vi "Traffic Monitoring Hub.vi"() -> ()   [LabVIEW 2018]
uses:
  TrafficMap/TrafficMap.lvclass
  <vilib>/LabVIEW Open Source Project/MQTT Broker/Client/Client.lvclass
  C:/Program Files (x86)/National Instruments/LabVIEW 2018/vi.lib/LabVIEW Open Source Project/MQTT Broker/MQTT_Base/MQTT_Base.lvclass
  <vilib>/LabVIEW Open Source Project/MQTT Broker/Control Packets/PUBLISH/PUBLISH.lvclass
  C:/Program Files (x86)/National Instruments/LabVIEW 2018/vi.lib/LabVIEW Open Source Project/MQTT Broker/Control Packets/ControlPacket/ControlPacket.lvclass
  typedefs/Node Type -- enum.ctl
  CarPool/CarPool.lvclass
  Zone/Zone.lvclass/Zone.ctl
  typedefs/RequestPayload -- cluster.ctl
  <vilib>/LabVIEW Open Source Project/MQTT Broker/Control Packets/ControlPacket/ControlPacket.lvclass/ControlPacket.ctl
  typedefs/ResponsePayload -- cluster.ctl
  TrafficMap/TrafficMap.lvclass/TrafficMap.ctl
  Car/Car State -- enum.ctl
  Car/Car.lvclass/Car.ctl
  Serializer.JKI-JSON/Serializer.JKI-JSON.lvclass
  C:/Program Files (x86)/National Instruments/LabVIEW 2018/vi.lib/LabVIEW Open Source Project/Serializer/Serializer/Serializer.lvclass
  <vilib>/LabVIEW Open Source Project/MQTT Broker/MQTT_Base/MQTT_Base.lvclass/MQTT_Base.ctl
  <vilib>/LabVIEW Open Source Project/MQTT Broker/Client/Client.lvclass/Client.ctl
  <vilib>/LabVIEW Open Source Project/MQTT Broker/Control Packets/CONNECT/ConnectFlags -- cluster.ctl
  typedefs/DisconnectPayload-- cluster.ctl
  typedefs/WillPayload -- cluster.ctl
  typedefs/ConnectPayload-- cluster.ctl
  82f4286b-0a94-4b9a-b9d4-821bcdb1e953.vi
  0d705227-134d-4031-8d1e-e35da49b8ba8.vi
  3d3687d4-2784-4a3f-94ff-e25152285f29.vi
  38838a55-6234-4be0-b764-729cd2a94195.vi
  e5968ec8-ddc8-4f80-9081-17407ede201a.vi
  bcdb7536-3eda-440d-b728-4c0836012992.vi
  bdf30a18-8ec8-4ac2-babb-b5048eb54a3e.vi
  3e129768-4a02-4394-80d2-37f91f557ee1.vi
  91350af8-47c3-4bac-a32d-49938f55f876.vi
  <vilib>/LabVIEW Open Source Project/Serializer/Serializer.FlattenedString/Serializer.FlattenedString.lvclass
  <vilib>/LabVIEW Open Source Project/MQTT Broker/MQTT_Base/Decode Publish Package.vi
  <vilib>/LabVIEW Open Source Project/Serializer/Serializer/Serializer.lvclass
  <vilib>/LabVIEW Open Source Project/MQTT Broker/MQTT_Base/MQTT_Base.lvclass
  <vilib>/LabVIEW Open Source Project/MQTT Broker/Control Packets/ControlPacket/ControlPacket.lvclass
  <vilib>/LabVIEW Open Source Project/MQTT Broker/Control Packets/CONNECT/CONNECT.lvclass
  <vilib>/addons/_JKI.lib/Serialization/JSON/JKI JSON Serialization.lvlib
  Car/Car.lvclass
  Zone/Zone.lvclass
  <vilib>/ptbypt/NI_PtbyPt.lvlib
panel:
  out "Zones":u32[](array[slide]) scale=0.0..11.4
  in  "# Cars":i32=1 min=1 max=20
  out "Message Frequency (Hz)":dbl
  out "error out":errorcluster
  out "Messages Processed":u32
  in  "Destroy Sim Cars":bool
  in  "Generate Sim Cars":bool
  out "Last Incoming Message":string
  out "Hub status":string
  out "Connection Status":string="Disconnected"
  out "Map":u16[][](graph)
  out "Zones":string[](array[string])
  in  "List Zones":bool
  out "Raw Packet String":string
  out "Payload":variant
  out "Topic":string
  # "Traffic Monitoring Hub"
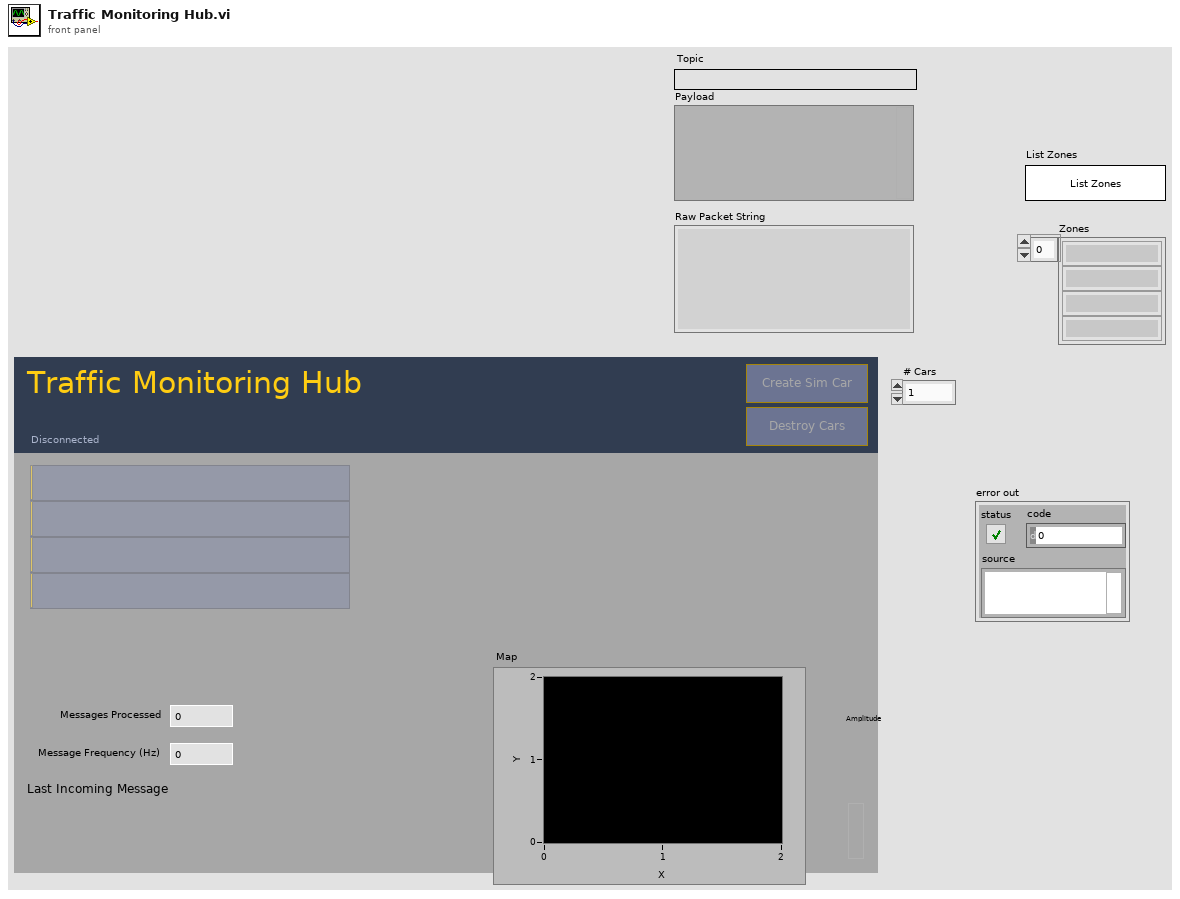
[diagram p1: front panel]
types:
  T1 = enum32{"Invalid", "Standard", "Closed", "Hidden", "Minimized", "Maximized"}
  T2 = enum32{"invalid app kind", "Development System", "Run Time System", "Student Edition", "Embedded LabVIEW", "Evaluation", "Custom"}
  T3 = typedef "RequestPayload -- cluster.ctl" = cluster{"request":string, "reply-to":string}
  T4 = typedef "ResponsePayload -- cluster.ctl" = cluster{"request":string, "reply":variant}
  T5 = typedef "Car.lvclass/Car State -- enum.ctl" = enum16{"parked", "driving"}
  T6 = typedef "CONNECT.lvclass/ConnectFlags -- cluster.ctl" = cluster{"Reserved":bool, "Clean Session":bool, "Will Flag":bool, "Will QoS 1":bool, "Will QoS 2":bool, "Will Retain":bool, "Password Flag":bool, "User Name Flag":bool}
  T7 = cluster{"Will Topic":string, "Will Message":string, "Username":string, "Password":string}
  T8 = typedef "DisconnectPayload-- cluster.ctl" = cluster{"timestamp":string}
  T9 = typedef "WillPayload -- cluster.ctl" = cluster{"message":string}
  T10 = typedef "ConnectPayload-- cluster.ctl" = cluster{"Node type":string}
  T11 = typedef "Node Type -- enum.ctl" = enum16{"Car", "Hub", "Sensor", "Relay"}
  T12 = cluster{"Core":cluster{"Current VI Reference":refnum<vi>, "Close Panel on Exit?":bool}, "server address":string, "project namespace":string, "Client Name":string, "Node type":T11, "Client":refnum<class "Client.lvclass">, "Close on MQTT Disconnection?":bool, "Subscription":string, "AppMessage":refnum<class "PUBLISH.lvclass">, "stop signal":refnum<user-event>, "TrafficMap":refnum<class "TrafficMap.lvclass">, "CarPool":refnum<class "CarPool.lvclass">, "Clones":string[]}
  T13 = cluster{"Current VI Reference":refnum<vi>, "Close Panel on Exit?":bool}
  T14 = cluster{"Messages Processed":u32, "seconds since 1Jan1904":timestamp}
  T15 = cluster{"Messages Processed":u32, "seconds since 1Jan1904":dbl}
  T16 = typedef "MQTT Server.lvlib/Client.lvclass/Public Events -- cluster.ctl" = cluster{"Connection Status":refnum<user-event>, "Connected":refnum<user-event>, "Application Message":refnum<user-event>}
  T17 = typedef "ControlPacket.lvclass/QualityOfService -- enum.ctl" = enum16{"0 (At Most Once)", "1 (At Least Once)", "2 (Exactly Once)"}
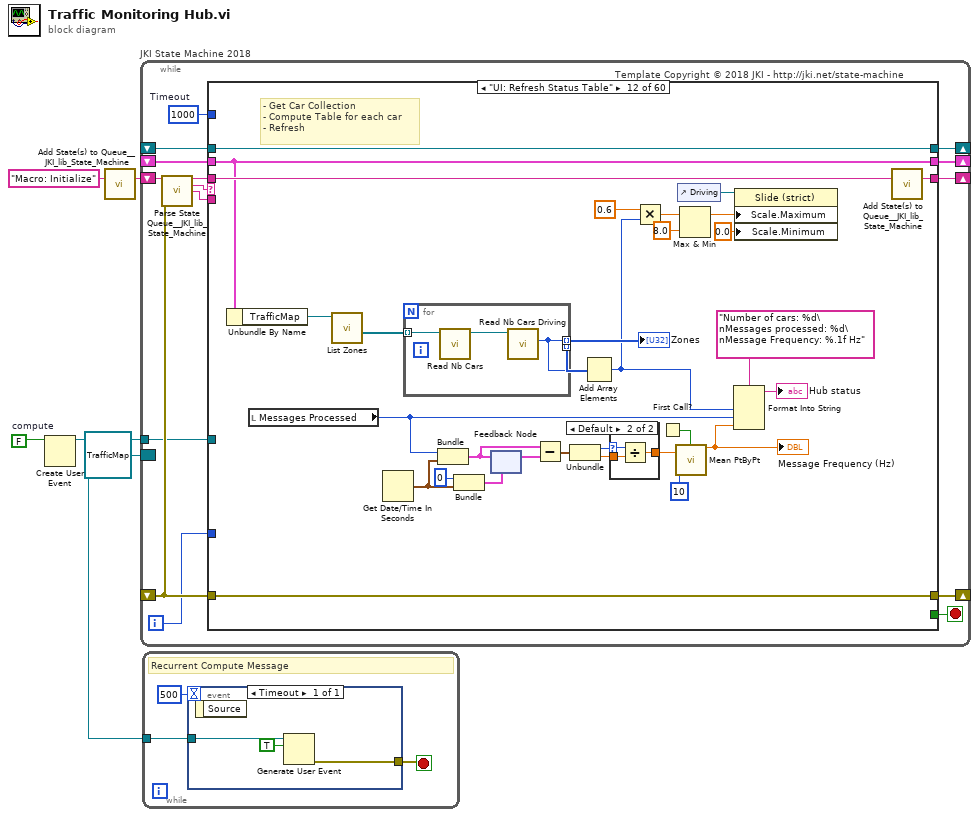
[diagram p0: block diagram]
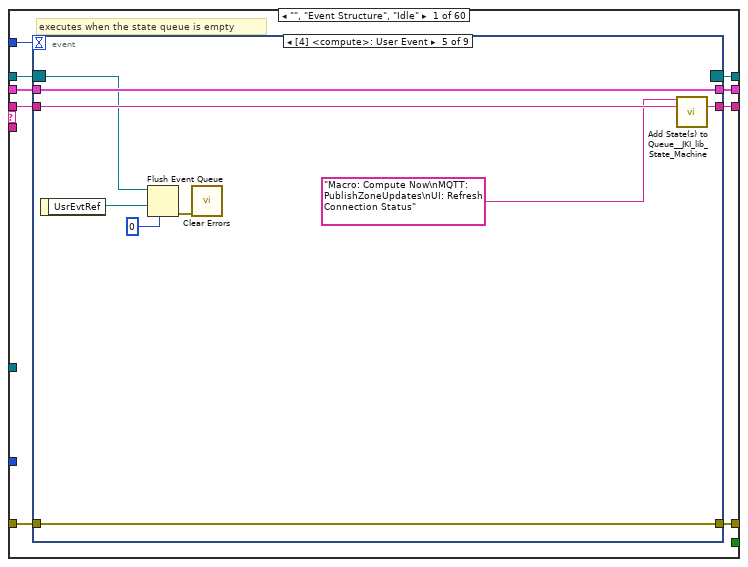
[diagram p2: hidden frame]
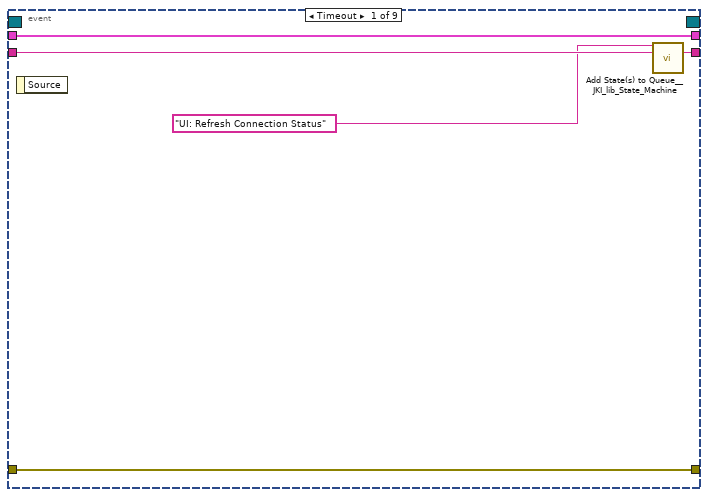
[diagram p3: hidden frame]
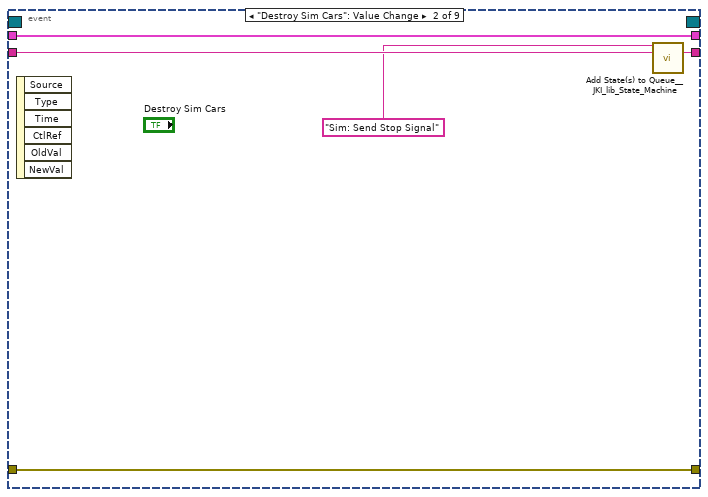
[diagram p4: hidden frame]
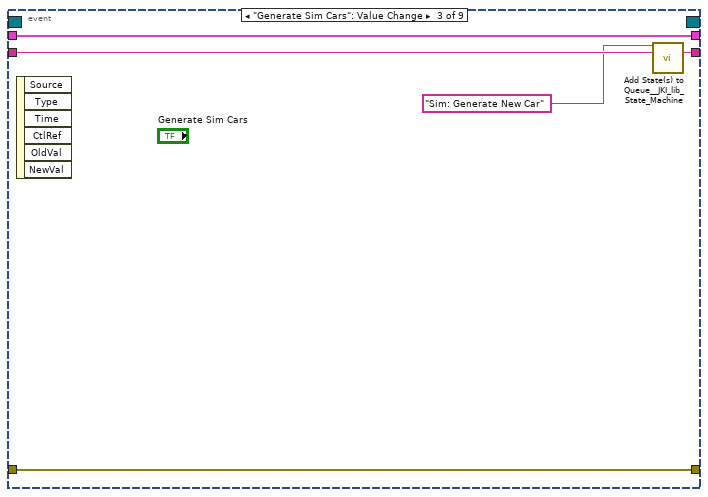
[diagram p5: hidden frame]
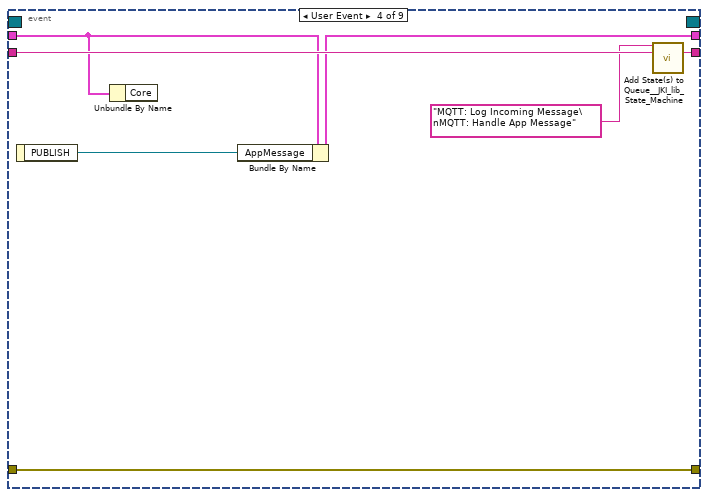
[diagram p6: hidden frame]
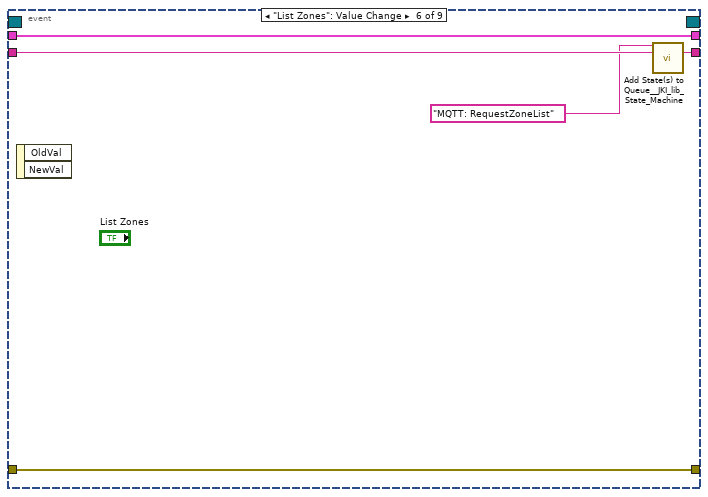
[diagram p7: hidden frame]
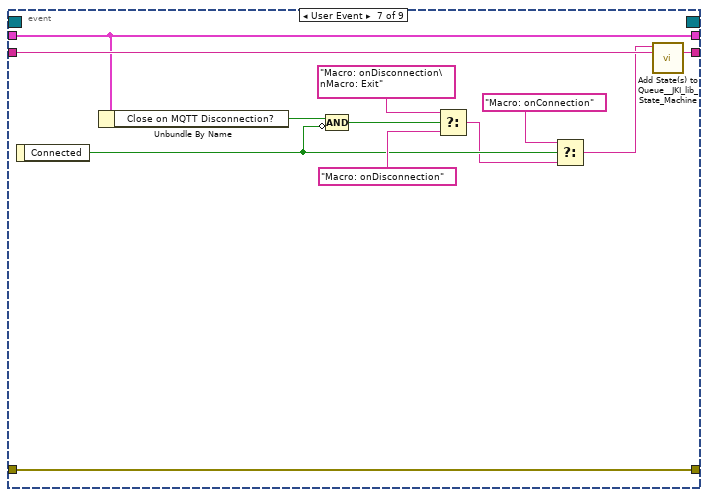
[diagram p8: hidden frame]
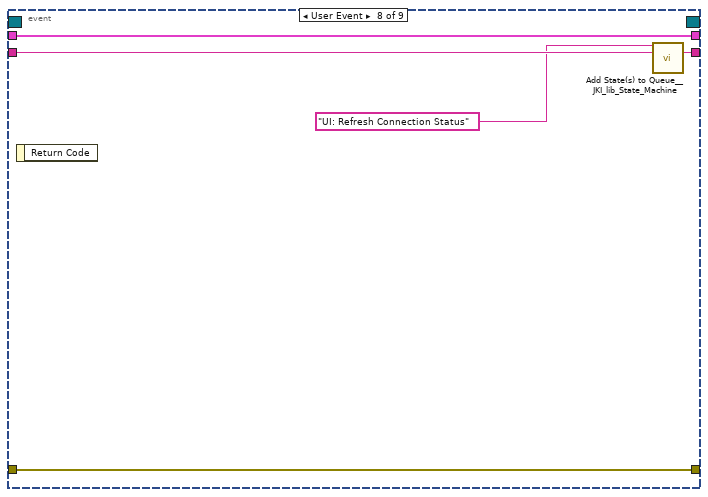
[diagram p9: hidden frame]
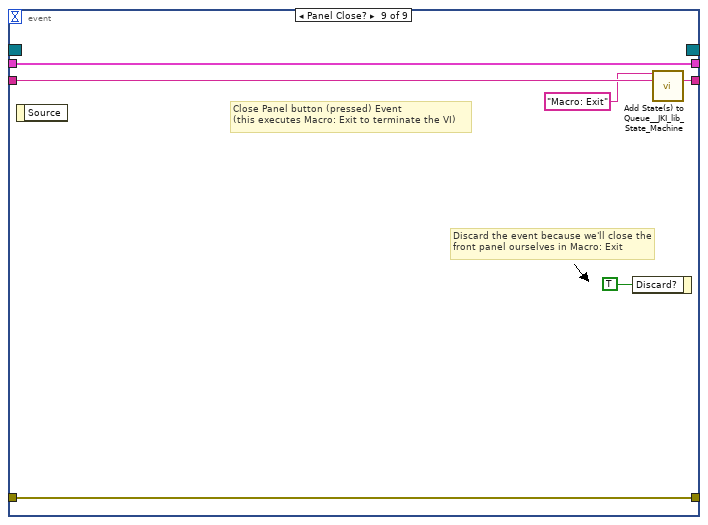
[diagram p10: hidden frame]
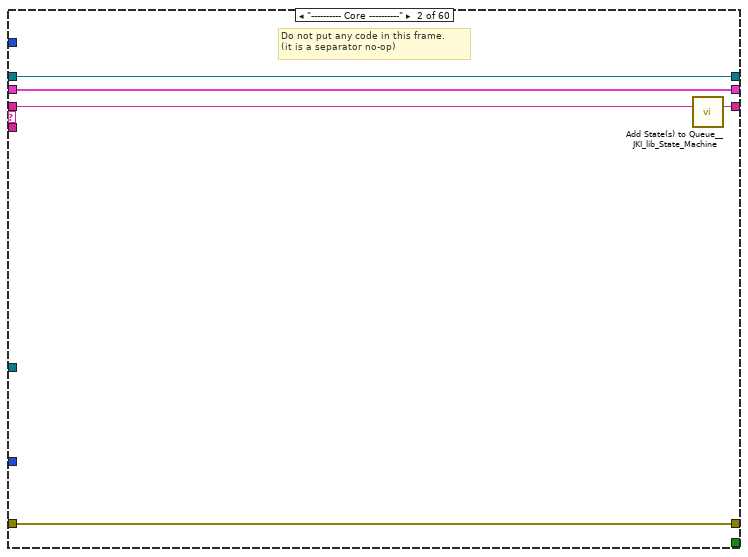
[diagram p11: hidden frame]
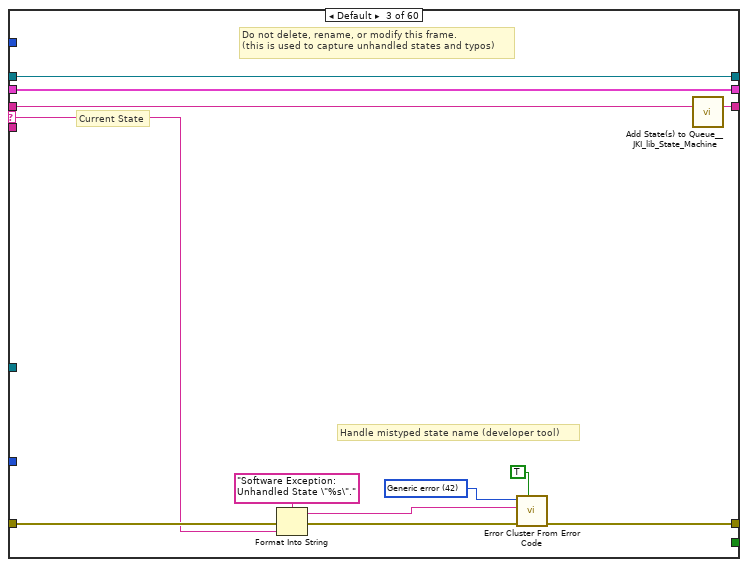
[diagram p12: hidden frame]
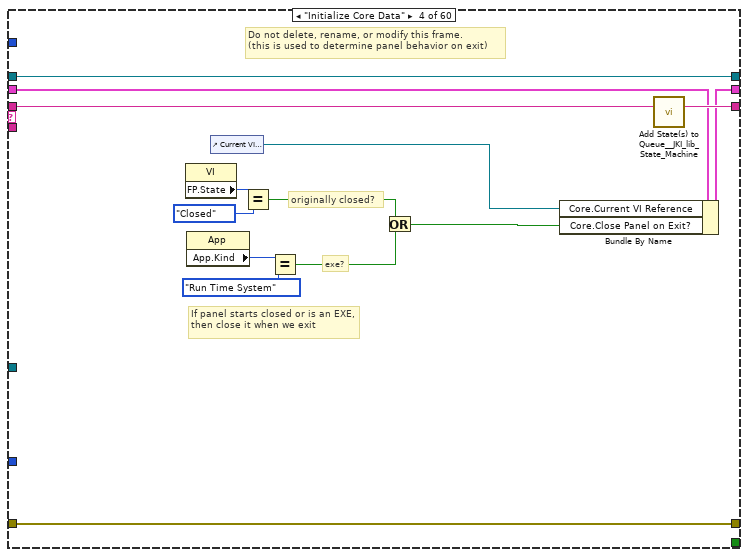
[diagram p13: hidden frame]
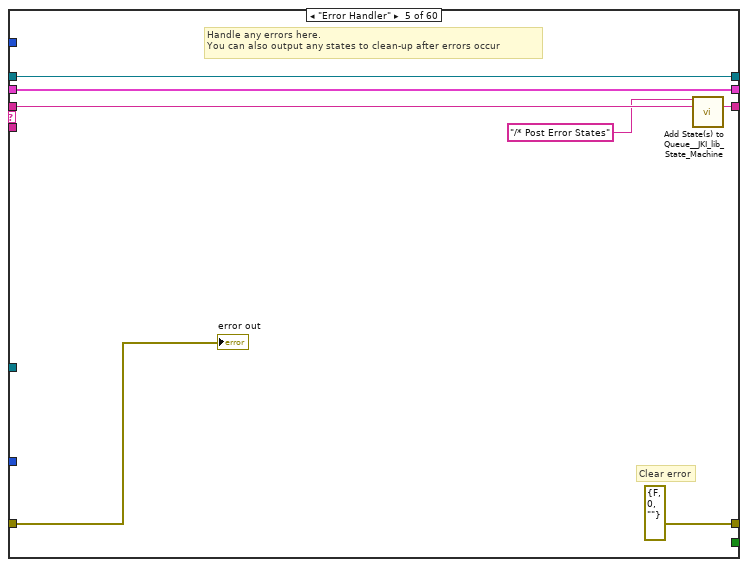
[diagram p14: hidden frame]
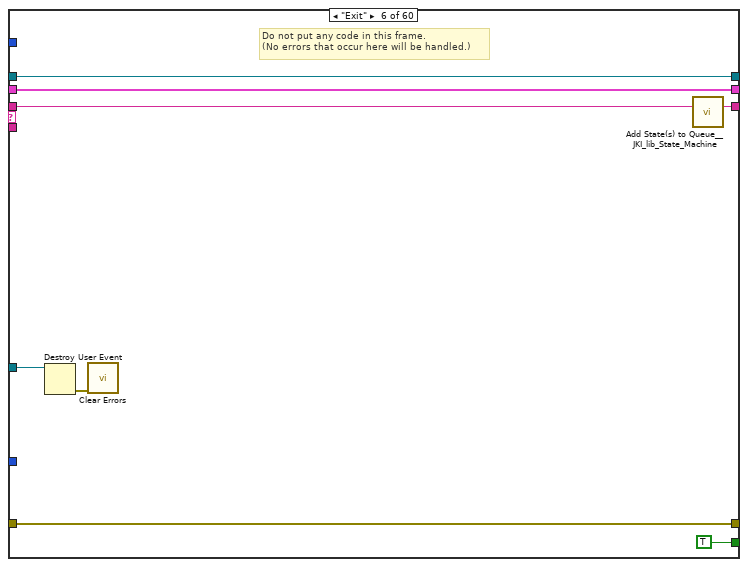
[diagram p15: hidden frame]
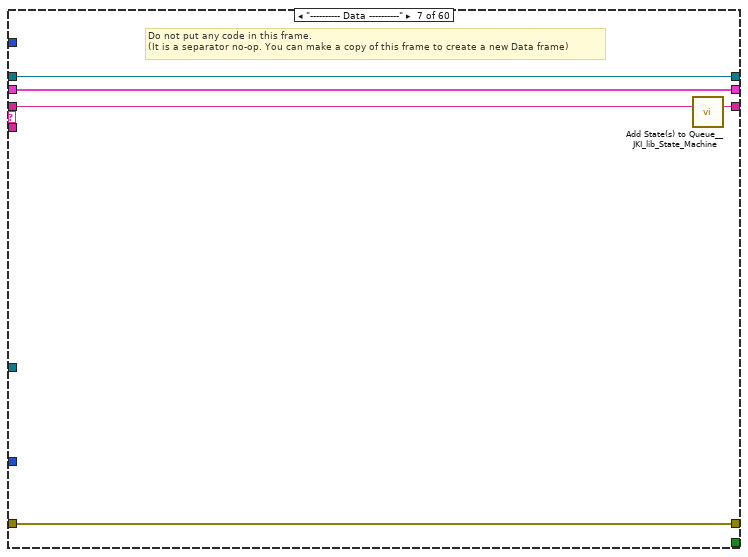
[diagram p16: hidden frame]
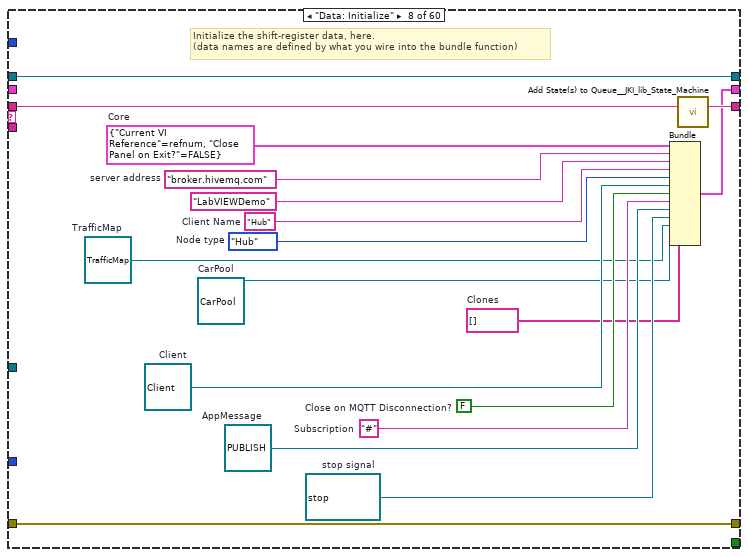
[diagram p17: hidden frame]
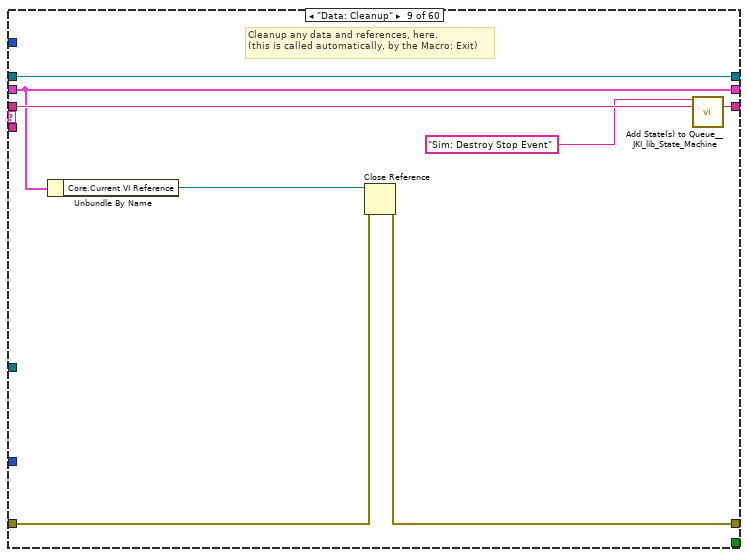
[diagram p18: hidden frame]
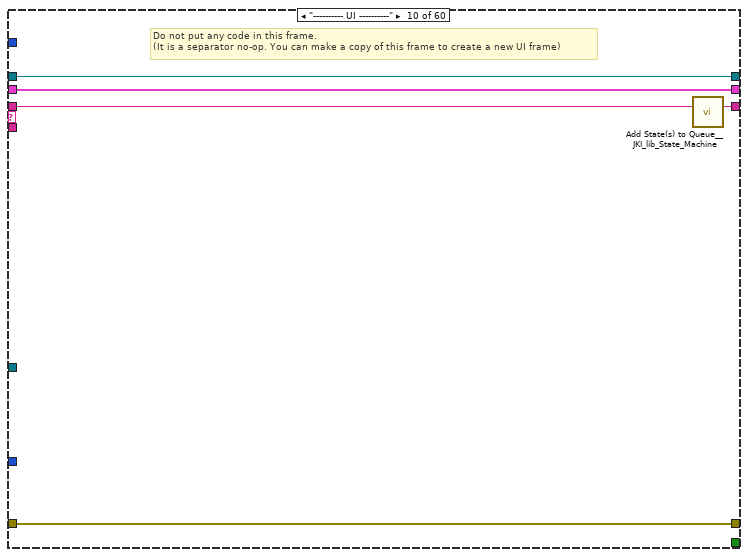
[diagram p19: hidden frame]
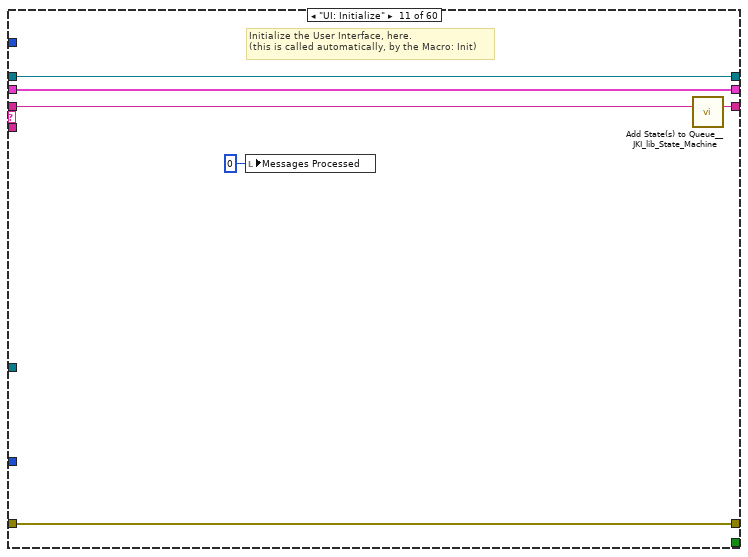
[diagram p20: hidden frame]
diagram:
  w3 = FALSE  # compute
  n1 = Create User Event(user event datatype=w3) -> (user event=w2:refnum<user-event>)  [unwired: 1 in, 1 out]
  n2 = call <vilib>:"Add State(s) to Queue__JKI_lib_State_Machine.vi"("State(s) in (\"\")"="Macro: Initialize") -> ("States Out"=w5:string)  [unwired: 14 in]
  n3 = while "JKI State Machine 2018" {
    shift-right: [w13] -> _
    shift-left: _ -> [w12]
    shift-right: [w16] -> _
    shift-left: _ -> [w10]
    shift-right: [w15] -> _
    shift-left: w5 -> [w17]
    shift-right: [w8] -> _
    shift-left: _ -> [w9]
    tunnel: w2 -> [w7]
    border: refnum<class "TrafficMap.lvclass"> refnum ("TrafficMap out") -> [_]
    i -> [w6]
    stop <- w14 stop-if-true
    w11 = 1000  # Timeout
    # "Template Copyright © 2018 JKI - http://jki.net/state-machine"
    n4 = call <vilib>:"Parse State Queue__JKI_lib_State_Machine.vi"("State Queue"=w17, "Error In (no error)"=w10) -> ("Remaining States"=w19:string, "Current State"=w20:string, "Arguments"=w18:string)  [unwired: 11 in]
    n5 = case shown="\"UI: Refresh Status Table\"" w20 {
      selector: w20 -> [_ _ w95 _ _ _ _ _ _ _ _ _ _ _ _ _ _ _ _ _ _ _ _ _ _ _ _ _ _ _ _ _ _ _ _ _ _ _ _ _ _ _ _ _ _ _ _ _ _ _ _ _ _ _ _ _ _ _ _ _]
      tunnel: w19 -> [w29 w93 w99 w119 w126 w134 w139 w157 w165 w170 w176 w207 w226 w233 w245 w315 w321 w327 w333 w339 w345 w351 w357 w363 w368 w374 w388 w393 w401 w407 w416 w431 w449 w466 w485 w493 w516 w540 w545 w557 w569 w593 w604 w617 w630 w644 w660 w724 w753 w779 w802 w817 w870 w884 w895 w926 w942 w953 w959 w966]
      tunnel: w18 -> [_ _ _ _ _ _ _ _ _ _ _ _ _ w228 w239 _ _ _ _ _ _ _ _ _ _ _ _ _ _ _ _ _ _ _ _ _ _ _ _ _ _ _ _ _ _ _ _ _ _ _ _ _ _ _ _ _ _ _ _ _]
      tunnel: w12 -> [w27 w90 w97 w112 w123 w132 w136 _ w160 w167 w174 w203 w216 w231 w241 w312 w318 w324 w330 w336 w342 w348 w354 w360 w365 w371 w385 w390 w395 w403 w410 w421 w446 w451 w482 w487 w511 w536 w542 w555 w566 w590 w597 w614 w627 w641 w645 w721 w750 w776 w799 w807 w867 w881 w888 w923 w939 w950 w954 w964]
      tunnel: [w26 w91 w101 w116 errorcluster {"status"=FALSE, "code"=0, "source"=""} ("error out") w131 w137 w154 w161 w168 w173 w205 w224 w229 w242 w313 w319 w325 w331 w337 w343 w349 w355 w361 w366 w372 w386 w391 w399 w405 w414 w429 w447 w460 w483 w491 w514 w538 w543 w547 w559 w584 w594 w606 w622 w632 w657 w719 w748 w774 w797 w814 w860 w874 w885 w914 w930 w945 w955 w961] -> w16
      tunnel: w10 -> [w25 w91 w100 w116 w120 w131 w137 w154 w162 w168 w173 w205 w224 w230 w243 w313 w319 w325 w331 w337 w343 w349 w355 w361 w366 w372 w386 w391 w399 w405 w414 w429 w447 w461 w483 w491 w514 w538 w543 w553 w562 w585 w595 w607 w623 w633 w657 w719 w748 w774 w797 w814 w861 w875 w886 w915 w931 w943 w956 w962]
      tunnel: [w28 w92 w98 w118 w125 w133 w138 w156 w164 w169 w175 w206 w225 w232 w244 w314 w320 w326 w332 w338 w344 w350 w356 w362 w367 w373 w387 w392 w400 w406 w415 w430 w448 w465 w484 w492 w515 w539 w544 w556 w568 w592 w603 w616 w629 w643 w659 w723 w752 w778 w801 w816 w869 w883 w894 w925 w941 w952 w958 w965] -> w15
      tunnel: [_ _ _ _ _ TRUE _ _ _ _ _ _ _ _ _ _ _ _ _ _ _ _ _ _ _ _ _ _ _ _ _ _ _ _ _ _ _ _ _ _ _ _ _ _ _ _ _ _ _ _ _ _ _ _ _ _ _ _ _ _] -> w14
      tunnel: [w24 w90 w97 w117 w123 w132 w136 w155 w160 w167 w174 w203 w216 w231 w241 w312 w318 w324 w330 w336 w342 w348 w354 w360 w365 w371 w385 w390 w394 w403 w409 w420 w446 w464 w482 w486 w510 w536 w542 w554 w567 w591 w597 w615 w628 w642 w645 w722 w751 w777 w800 w807 w868 w882 w888 w924 w940 w951 w954 w964] -> w13
      tunnel: w11 -> [w23 _ _ _ _ _ _ _ _ _ _ _ _ _ _ _ _ _ _ _ _ _ _ _ _ _ _ _ _ _ _ _ _ _ _ _ _ _ _ _ _ _ _ _ _ _ _ _ _ _ _ _ _ _ _ _ _ _ _ _]
      tunnel: w9 -> [w22 w89 w94 w106 w121 w129 w135 w148 w159 w166 w172 w204 w223 w227 w238 w311 w316 w322 w328 w334 w340 w346 w352 w358 w364 w369 w377 w389 w398 w404 w413 w428 w445 w463 w481 w490 w513 w537 w541 w552 _ w589 w602 w613 w626 w640 w658 w720 w749 w775 w798 w815 w866 w880 w893 w922 w938 w949 w957 w960]
      tunnel: [w21 w89 w94 w106 w121 w129 w135 w148 w159 w166 w172 w204 w223 w227 w238 w311 w316 w322 w328 w334 w340 w346 w352 w358 w364 w369 w377 w389 w398 w404 w413 w428 w445 w463 w481 w490 w513 w537 w541 w552 w561 w589 w602 w613 w626 w640 w658 w720 w749 w775 w798 w815 w866 w880 w893 w922 w938 w949 w957 w960] -> w8
      tunnel: w7 -> [_ _ _ _ _ w128 _ _ _ _ _ _ _ _ _ _ _ _ _ _ _ _ _ _ _ _ w375 _ _ _ _ _ _ _ _ _ _ _ _ _ w558 _ _ _ _ _ _ _ _ _ _ _ _ _ _ _ _ _ _ _]
      tunnel: w6 -> [_ _ _ _ _ _ _ _ _ _ _ _ _ _ _ _ _ _ _ _ _ _ _ _ _ _ _ _ _ _ _ _ _ _ _ _ w500 _ _ _ _ _ _ _ _ _ _ _ _ _ _ _ _ _ _ _ _ _ _ _]
      frame "", "Event Structure", "Idle" {
        # "executes when the state queue is empty"
        n6 = event shown="[4] <compute>: User Event" {
          selector: w22 -> [_ _ _ _ w55 _ _ _ _]
          dyn-events: [_ _ _ _ _ _ _ _ _] -> w21
          timeout: w23 -> [_ _ _ _ _ _ _ _ _]
          tunnel: w29 -> [w34 w39 w44 w51 w60 w65 w77 w82 w88]
          tunnel: [w33 w38 w43 w50 w59 w64 w76 w81 w87] -> w28
          tunnel: w27 -> [w32 w36 w41 w47 w56 w61 w74 w79 w85]
          tunnel: [w31 w37 w42 w49 w58 w63 w75 w80 w86] -> w26
          tunnel: w25 -> [w31 w37 w42 w49 w58 w63 w75 w80 w86]
          tunnel: [w32 w36 w41 w46 w56 w61 w74 w79 w85] -> w24
          event Timeout {
            n7 = event-data() -> ()  [unwired: 1 in, 1 out]
            n8 = call <vilib>:"Add State(s) to Queue__JKI_lib_State_Machine.vi"("State(s) in Front (\"\")"="UI: Refresh Connection Status", "State(s) in (\"\")"=w34) -> ("States Out"=w33:string)  [unwired: 13 in]
          }
          event "Destroy Sim Cars": Value Change {
            n9 = event-data() -> ()  [unwired: 1 in, 6 out]
            n10 = call <vilib>:"Add State(s) to Queue__JKI_lib_State_Machine.vi"("State(s) in Front (\"\")"="Sim: Send Stop Signal", "State(s) in (\"\")"=w39) -> ("States Out"=w38:string)  [unwired: 13 in]
          }
          event "Generate Sim Cars": Value Change {
            n11 = event-data() -> ()  [unwired: 1 in, 6 out]
            n12 = call <vilib>:"Add State(s) to Queue__JKI_lib_State_Machine.vi"("State(s) in Front (\"\")"="Sim: Generate New Car", "State(s) in (\"\")"=w44) -> ("States Out"=w43:string)  [unwired: 13 in]
          }
          event User Event {
            n13 = event-data() -> ("PUBLISH"=w48:refnum<class "PUBLISH.lvclass">)  [unwired: 1 in]
            n14 = Unbundle By Name(w47) -> ()  [unwired: 1 out]
            n15 = Bundle By Name(cluster=w47, "AppMessage"=w48) -> (w46:T12)
            n16 = call <vilib>:"Add State(s) to Queue__JKI_lib_State_Machine.vi"("State(s) in Front (\"\")"="MQTT: Log Incoming Message\nMQTT: Handle App Message", "State(s) in (\"\")"=w51) -> ("States Out"=w50:string)  [unwired: 13 in]
          }
          event User Event {
            n17 = event-data() -> ("UsrEvtRef"=w54:refnum<user-event>)  [unwired: 1 in]
            n18 = Flush Event Queue(0:w55, 2:w54, 5:0 ("keep most recent")) -> (11:w52:errorcluster)  [unwired: 3 in, 2 out]
            n19 = call <vilib>:"Clear Errors.vi"("error in (no error)"=w52) -> ()  [unwired: 5 in, 2 out]
            n20 = call <vilib>:"Add State(s) to Queue__JKI_lib_State_Machine.vi"("State(s) in Front (\"\")"="Macro: Compute Now\nMQTT: PublishZoneUpdates\nUI: Refresh Connection Status", "State(s) in (\"\")"=w60) -> ("States Out"=w59:string)  [unwired: 13 in]
          }
          event "List Zones": Value Change {
            n21 = event-data() -> ()  [unwired: 1 in, 2 out]
            n22 = call <vilib>:"Add State(s) to Queue__JKI_lib_State_Machine.vi"("State(s) in Front (\"\")"="MQTT: RequestZoneList", "State(s) in (\"\")"=w65) -> ("States Out"=w64:string)  [unwired: 13 in]
          }
          event User Event {
            n23 = event-data() -> ("Connected"=w69:bool)  [unwired: 1 in]
            n24 = Unbundle By Name(w74) -> ("Close on MQTT Disconnection?"=w73:bool)
            n25 = Compound Arithmetic op=AND(w73, invert w69) -> (w72:bool)
            n26 = Select(t="Macro: onDisconnection\nMacro: Exit", s=w72, f="Macro: onDisconnection" ("t")) -> (s? t:f=w67:string)
            n27 = Select(t="Macro: onConnection", s=w69, f=w67) -> (s? t:f=w66:string)
            n28 = call <vilib>:"Add State(s) to Queue__JKI_lib_State_Machine.vi"("State(s) in Front (\"\")"=w66, "State(s) in (\"\")"=w77) -> ("States Out"=w76:string)  [unwired: 13 in]
          }
          event User Event {
            n29 = event-data() -> ()  [unwired: 1 in, 1 out]
            n30 = call <vilib>:"Add State(s) to Queue__JKI_lib_State_Machine.vi"("State(s) in Front (\"\")"="UI: Refresh Connection Status", "State(s) in (\"\")"=w82) -> ("States Out"=w81:string)  [unwired: 13 in]
          }
          event Panel Close? {
            # "Discard the event because we'll close the front panel ourselves in Macro: Exit"
            # "Close Panel button (pressed) Event\n(this executes Macro: Exit to terminate the VI)"
            n31 = event-data() -> ()  [unwired: 1 in, 1 out]
            n32 = event-data("Discard?"=TRUE) -> ()  [unwired: 1 in, 1 out]
            n33 = call <vilib>:"Add State(s) to Queue__JKI_lib_State_Machine.vi"("State(s) in Front (\"\")"="Macro: Exit", "State(s) in (\"\")"=w88) -> ("States Out"=w87:string)  [unwired: 13 in]
          }
        }
      }
      frame "---------- Core ----------" {
        # "Do not put any code in this frame.\n(it is a separator no-op)"
        n34 = call <vilib>:"Add State(s) to Queue__JKI_lib_State_Machine.vi"("State(s) in (\"\")"=w93) -> ("States Out"=w92:string)  [unwired: 14 in]
      }
      frame Default {
        w104 = 42 items=["No error", "Argument error", "Memory is full", "Out of zone", "End of file", "File already open", "Generic file I/O error", "File not found", "File permission error", "Disk is full", "Duplicate path", "Too many files open", "System feature not enabled", "Resource file not found", "Cannot add resource", "Resource not found", "Image not found", "Image memory error", "Pen does not exist", "Config type invalid", "Config token not found", "Config parse error", "Config memory error", "Bad external code format", "Bad external code offset", "External code not present", "Null window", "Destroy window error", "Null menu", "Print aborted", "Bad print record", "Print driver error", "Windows error during printing", "Memory error during printing", "Print dialog error", "Generic print error", "Invalid device refnum", "Device not found", "Device parameter error", "Device unit error", "Cannot open device", "Device call aborted", "Generic error", "Cancelled by user", "Object ID too low", "Object ID too high", "Object not in heap", "Unknown heap", "Unknown object (invalid DefProc)", "Unknown object (DefProc not in table)", "Message out of range", "Invalid (null) method", "Unknown message", "Manager call not supported", "Bad address", "Network operation in progress", "Network operation timed out", "Connection is busy", "Network attribute not supported", "Network error", "Address in use", "System out of memory", "Connection aborted", "Connection refused", "Not connected", "Already connected", "Connection closed", "Initialization error (interapplication manager)", "Bad occurrence", "Wait on unbound occurrence handler", "Occurrence queue overflow", "Datalog type conflict", "Unused", "Unrecognized type (interapplication manager)", "Memory corrupt", "Failed to make temporary DLL", "Old CIN version", "Drag socket not found", "Failed to load drop-object", "Failed to register OLE object", "Failed to release OLE object", "Format specifier type mismatch", "Unknown format specifier", "Too few format specifiers", "Too many format specifiers", "Scan failed", "Newer CIN version", "Error converting to variant", "Runtime menu error", "Password tampered", "Variant attribute not found", "Incompatible variant data type", "Event data is not available", "Event Store is not present", "Occurrence is not found", "Event Queue is not created", "Event info is not available", "Refnum passed is NULL", "Error retrieving Class GUID", "Error retrieving CoClass GUID", "Error retrieving TypeLib GUID.", "Bad built application magic bytes.", "Specific driver is different from the specific driver associated with the Logical Name.", "There is no session opened to the class driver.", "Max Error", "MAX - Error with config objects", "MAX - Error loading configuration", "MAX - Group not supported"]
        # "Current State"
        # "Do not delete, rename, or modify this frame.\n(this is used to capture unhandled states and typos)"
        # "Handle mistyped state name (developer tool)"
        n35 = Format Into String(format string="Software Exception: Unhandled State \"%s\"." ("message"), error in=w100, w95) -> (resulting string=w103:string, error out=w102:errorcluster)  [unwired: 1 in]
        n36 = call <vilib>:"Error Cluster From Error Code.vi"("show call chain? (False)"=TRUE, "error in (no error)"=w102, "error message (\"\")"=w103, "error code (0)"=w104) -> ("error out"=w101:errorcluster)  [unwired: 5 in]
        n37 = call <vilib>:"Add State(s) to Queue__JKI_lib_State_Machine.vi"("State(s) in (\"\")"=w99) -> ("States Out"=w98:string)  [unwired: 14 in]
      }
      frame "Initialize Core Data" {
        # "Do not delete, rename, or modify this frame.\n(this is used to determine panel behavior on exit)"
        # "originally closed?"
        # "exe?"
        # "If panel starts closed or is an EXE, then close it when we exit"
        n38 = property class="VI"() -> ("FP.State"=w109:T1)  [unwired: 2 in, 2 out]
        n39 = property class="App"() -> ("App.Kind"=w115:T2)  [unwired: 2 in, 2 out]
        n40 = control-ref of="Current VI Reference"() -> (w110:refnum<vi>)
        n41 = Equal?(x=w109, y=T1."Closed" ("Front Panel Window:State")) -> (x = y?=w107:bool)
        n42 = Equal?(x=w115, y=T2."Run Time System" ("Application:Kind")) -> (x = y?=w113:bool)
        n43 = Or(x=w107, y=w113) -> (x .or. y?=w111:bool)
        n44 = Bundle By Name(cluster=w112, "Core.Current VI Reference"=w110, "Core.Close Panel on Exit?"=w111) -> (w117:T12)
        n45 = call <vilib>:"Add State(s) to Queue__JKI_lib_State_Machine.vi"("State(s) in (\"\")"=w119) -> ("States Out"=w118:string)  [unwired: 14 in]
      }
      frame "Error Handler" {
        # "Handle any errors here.\nYou can also output any states to clean-up after errors occur"
        # "Clear error"
        n46 = call <vilib>:"Add State(s) to Queue__JKI_lib_State_Machine.vi"("State(s) in Front (\"\")"="/* Post Error States", "State(s) in (\"\")"=w126) -> ("States Out"=w125:string)  [unwired: 13 in]
        "error out" <- w120
      }
      frame "Exit" {
        # "Do not put any code in this frame.\n(No errors that occur here will be handled.)"
        n47 = Destroy User Event(user event=w128) -> (error out=w127:errorcluster)  [unwired: 1 in]
        n48 = call <vilib>:"Clear Errors.vi"("error in (no error)"=w127) -> ()  [unwired: 5 in, 2 out]
        n49 = call <vilib>:"Add State(s) to Queue__JKI_lib_State_Machine.vi"("State(s) in (\"\")"=w134) -> ("States Out"=w133:string)  [unwired: 14 in]
      }
      frame "---------- Data ----------" {
        # "Do not put any code in this frame.\n(It is a separator no-op. You can make a copy of this frame to create a new Data frame)"
        n50 = call <vilib>:"Add State(s) to Queue__JKI_lib_State_Machine.vi"("State(s) in (\"\")"=w139) -> ("States Out"=w138:string)  [unwired: 14 in]
      }
      frame "Data: Initialize" {
        w140 = string[] []  # Clones
        w141 = refnum<class "CarPool.lvclass"> refnum  # CarPool
        w142 = refnum<class "TrafficMap.lvclass"> refnum  # TrafficMap
        w143 = Node_Type_--_enum."Hub"  # Node type
        w144 = refnum<user-event> refnum  # stop signal
        w145 = refnum<class "PUBLISH.lvclass"> refnum  # AppMessage
        w146 = "#"  # Subscription
        w147 = FALSE  # Close on MQTT Disconnection?
        w149 = refnum<class "Client.lvclass"> refnum  # Client
        w150 = "broker.hivemq.com"  # server address
        w152 = T13 {"Current VI Reference"=refnum, "Close Panel on Exit?"=FALSE}  # Core
        w153 = "Hub"  # Client Name
        # "Initialize the shift-register data, here.\n(data names are defined by what you wire into the bundle function)"
        n51 = Bundle("Core"=w152, "server address"=w150, "project namespace"="LabVIEWDemo", "Client Name"=w153, "Node type"=w143, "Client"=w149, "Close on MQTT Disconnection?"=w147, "Subscription"=w146, "AppMessage"=w145, "stop signal"=w144, "TrafficMap"=w142, "CarPool"=w141, "Clones"=w140) -> (w155:T12)  [unwired: 1 in]
        n52 = call <vilib>:"Add State(s) to Queue__JKI_lib_State_Machine.vi"("State(s) in (\"\")"=w157) -> ("States Out"=w156:string)  [unwired: 14 in]
      }
      frame "Data: Cleanup" {
        # "Cleanup any data and references, here.\n(this is called automatically, by the Macro: Exit)"
        n53 = Unbundle By Name(w160) -> ("Core.Current VI Reference"=w163:refnum<vi>)
        n54 = Close Reference(reference=w163, error in (no error)=w162) -> (error out=w161:errorcluster)
        n55 = call <vilib>:"Add State(s) to Queue__JKI_lib_State_Machine.vi"("State(s) in Front (\"\")"="Sim: Destroy Stop Event", "State(s) in (\"\")"=w165) -> ("States Out"=w164:string)  [unwired: 13 in]
      }
      frame "---------- UI ----------" {
        # "Do not put any code in this frame.\n(It is a separator no-op. You can make a copy of this frame to create a new UI frame)"
        n56 = call <vilib>:"Add State(s) to Queue__JKI_lib_State_Machine.vi"("State(s) in (\"\")"=w170) -> ("States Out"=w169:string)  [unwired: 14 in]
      }
      frame "UI: Initialize" {
        # "Initialize the User Interface, here.\n(this is called automatically, by the Macro: Init)"
        n57 = local write "Messages Processed"(u32 0 ("Messages Processed")) -> ()
        n58 = call <vilib>:"Add State(s) to Queue__JKI_lib_State_Machine.vi"("State(s) in (\"\")"=w176) -> ("States Out"=w175:string)  [unwired: 14 in]
      }
      frame "UI: Refresh Status Table" {
        # "- Get Car Collection\n- Compute Table for each car\n- Refresh"
        n59 = Unbundle By Name(w203) -> ("TrafficMap"=w202:refnum<class "TrafficMap.lvclass">)
        n60 = local read "Messages Processed"() -> (w187:u32)
        n61 = call "List Zones.vi"("TrafficMap in"=w202) -> ("Instances"=w201:refnum<class "Zone.lvclass">[])  [unwired: 7 in, 3 out]
        n62 = Get Date/Time In Seconds() -> (seconds since 1Jan1904=w197:timestamp)
        n63 = for {
          tunnel: w201 -> [w214] mode=indexing
          tunnel: [w212] -> w200 mode=indexing
          tunnel: [w212] -> w185 mode=indexing
          n64 = call "Read Nb Cars.vi"("Zone in"=w214) -> ("Zone out"=w213:refnum<class "Zone.lvclass">)  [unwired: 8 in, 2 out]
          n65 = call "Read Nb Cars Driving.vi"("Zone in"=w213) -> ("Nb Cars Driving"=w212:u32)  [unwired: 8 in, 2 out]
        }
        "Zones" <- w185
        n66 = Bundle("Messages Processed"=w187, "seconds since 1Jan1904"=w197) -> (w193:T14)  [unwired: 1 in]
        n67 = Bundle("Messages Processed"=u32 0, "seconds since 1Jan1904"=w197) -> (w195:T14)  [unwired: 1 in]
        n68 = feedback-in #1(w193) -> ()
        n69 = feedback #1(w195) -> (w194:T14)
        n70 = Subtract(x=w193, y=w194) -> (x-y=w192:T15)
        n71 = Unbundle(w192) -> ("Messages Processed"=w182:u32, "seconds since 1Jan1904"=w191:dbl)
        n72 = Add Array Elements(numeric array=w200) -> (sum=w183:u32)
        n73 = case shown="Default" w182 {
          selector: w182 -> [w208 w209]
          tunnel: w191 -> [_ w211]
          tunnel: [w208 w210] -> w181
          frame 0 {
          }
          frame Default {
            n74 = Divide(x=w209, y=w211) -> (x/y=w210:dbl)
          }
        }
        n75 = Multiply(x=0.6, y=w183) -> (x*y=w179:dbl)
        n76 = First Call?() -> (First Call?: T/F=w177:bool)
        n77 = call <vilib>:"Mean PtByPt.vi"("x"=w181, "sample length"=10, "initialize"=w177) -> ("mean"=w186:dbl)  [unwired: 1 in, 1 out]
        "Message Frequency (Hz)" <- w186
        n78 = control-ref of="Driving"() -> (w188:refnum<vi>)
        n79 = Max & Min(x=w179, y=8.0) -> (max(x,y)=w178:dbl)  [unwired: 1 out]
        n80 = Format Into String(format string="Number of cars: %d\nMessages processed: %d\nMessage Frequency: %.1f Hz", w183, w187, w186) -> (resulting string=→"Hub status":string)  [unwired: 2 in, 1 out]
        n81 = property on="Property Node" class="Slide (strict)"(reference=w188, "Scale.Maximum"=w178, "Scale.Minimum"=0.0 ("Scale.Range:Minimum")) -> ()  [unwired: 1 in, 2 out]
        n82 = call <vilib>:"Add State(s) to Queue__JKI_lib_State_Machine.vi"("State(s) in (\"\")"=w207) -> ("States Out"=w206:string)  [unwired: 14 in]
      }
      frame "UI: Refresh Connection Status" {
        n83 = Unbundle By Name(w216) -> ("Client"=w222:refnum<class "Client.lvclass">, "server address"=w218:string)
        n84 = call <vilib>:"isConnected.vi"("Client in"=w222) -> ("connected"=w221:bool)  [unwired: 8 in, 2 out]
        n85 = Format Into String("Connected", w218) -> (resulting string=w217:string)  [unwired: 3 in, 1 out]
        n86 = Select(t=w217, s=w221, f="Disconnected") -> (s? t:f=→"Connection Status":string)
        n87 = call <vilib>:"Add State(s) to Queue__JKI_lib_State_Machine.vi"("State(s) in (\"\")"=w226) -> ("States Out"=w225:string)  [unwired: 14 in]
      }
      frame "UI: Cursor Set" {
        # "Argument"
        # "Set and Unset Cursor Busy.\n(Usage: \"UI: Cursor Set >> Busy|Idle\")"
        n88 = case shown="\"Idle\", Default" w228 {
          tunnel: w230 -> [w235 w237]
          tunnel: [w234 w236] -> w229
          frame "Idle", Default {
            n89 = call <vilib>:"Unset Busy.vi"("error in (no error)"=w235) -> ("error out"=w234:errorcluster)  [unwired: 10 in]
          }
          frame "Busy" {
            n90 = call <vilib>:"Set Busy.vi"("error in (no error)"=w237) -> ("error out"=w236:errorcluster)  [unwired: 9 in, 1 out]
          }
        }
        n91 = call <vilib>:"Add State(s) to Queue__JKI_lib_State_Machine.vi"("State(s) in (\"\")"=w233) -> ("States Out"=w232:string)  [unwired: 14 in]
      }
      frame "UI: Front Panel State" {
        # "Argument"
        # "Set Front Panel Open or Closed\n(Usage: \"UI: Front Panel State >> Open|Close\")"
        n92 = Unbundle By Name(w241) -> ("Core.Current VI Reference"=w240:refnum<vi>)
        n93 = case shown="\"Minimize\", \"Minimized\"" w239 {
          tunnel: w243 -> [w251 w266 w277 w290 w303]
          tunnel: [w253 w267 w279 w292 w305] -> w242
          tunnel: w240 -> [w252 w264 w278 w291 w304]
          frame "Open", "Standard", Default {
            w246 = T1."Standard" ("State")
            n94 = property class="VI"(reference=w252, error in=w251) -> (reference out=w249:refnum<vi>, error out=w250:errorcluster, "FP.State"=w248:T1)
            n95 = Not Equal?(x=w248, y=w246) -> (x != y?=w247:bool)
            n96 = case shown="True" w247 {
              tunnel: [w257 w259] -> w253
              tunnel: w250 -> [w256 w259]
              tunnel: w249 -> [w255 _]
              tunnel: w246 -> [w254 _]
              frame True {
                n97 = invoke class="VI" method="FP.Open"(reference=w255, error in=w256, "Activate"=TRUE, "State"=w254) -> (error out=w257:errorcluster)  [unwired: 1 in, 4 out]
              }
              frame False {
              }
            }
          }
          frame "Close", "Closed" {
            n98 = property class="VI"(reference=w264, error in=w266) -> (reference out=w263:refnum<vi>, error out=w265:errorcluster, "FP.State"=w261:T1)
            n99 = Not Equal?(x=w261, y=T1."Closed" ("Front Panel Window:State")) -> (x != y?=w260:bool)
            n100 = case shown="True" w260 {
              tunnel: [w268 w271] -> w267
              tunnel: w265 -> [w268 w270]
              tunnel: w263 -> [_ w269]
              frame False {
              }
              frame True {
                n101 = invoke class="VI" method="FP.Close"(reference=w269, error in=w270) -> (error out=w271:errorcluster)  [unwired: 1 in, 2 out]
              }
            }
          }
          frame "Hidden", "Hide" {
            w272 = T1."Hidden" ("State")
            n102 = property class="VI"(reference=w278, error in=w277) -> (reference out=w275:refnum<vi>, error out=w276:errorcluster, "FP.State"=w274:T1)
            n103 = Not Equal?(x=w274, y=w272) -> (x != y?=w273:bool)
            n104 = case shown="True" w273 {
              tunnel: [w283 w284] -> w279
              tunnel: w276 -> [w282 w284]
              tunnel: w275 -> [w281 _]
              tunnel: w272 -> [w280 _]
              frame True {
                n105 = invoke class="VI" method="FP.Open"(reference=w281, error in=w282, "State"=w280) -> (error out=w283:errorcluster)  [unwired: 2 in, 4 out]
              }
              frame False {
              }
            }
          }
          frame "Minimize", "Minimized" {
            w285 = T1."Minimized" ("State")
            n106 = property class="VI"(reference=w291, error in=w290) -> (reference out=w288:refnum<vi>, error out=w289:errorcluster, "FP.State"=w287:T1)
            n107 = Not Equal?(x=w287, y=w285) -> (x != y?=w286:bool)
            n108 = case shown="True" w286 {
              tunnel: [w296 w297] -> w292
              tunnel: w289 -> [w295 w297]
              tunnel: w288 -> [w294 _]
              tunnel: w285 -> [w293 _]
              frame True {
                n109 = invoke class="VI" method="FP.Open"(reference=w294, error in=w295, "State"=w293) -> (error out=w296:errorcluster)  [unwired: 2 in, 4 out]
              }
              frame False {
              }
            }
          }
          frame "Maximize", "Maximized" {
            w298 = T1."Maximized" ("State")
            n110 = property class="VI"(reference=w304, error in=w303) -> (reference out=w301:refnum<vi>, error out=w302:errorcluster, "FP.State"=w300:T1)
            n111 = Not Equal?(x=w300, y=w298) -> (x != y?=w299:bool)
            n112 = case shown="True" w299 {
              tunnel: [w309 w310] -> w305
              tunnel: w302 -> [w308 w310]
              tunnel: w301 -> [w307 _]
              tunnel: w298 -> [w306 _]
              frame True {
                n113 = invoke class="VI" method="FP.Open"(reference=w307, error in=w308, "State"=w306) -> (error out=w309:errorcluster)  [unwired: 2 in, 4 out]
              }
              frame False {
              }
            }
          }
        }
        n114 = call <vilib>:"Add State(s) to Queue__JKI_lib_State_Machine.vi"("State(s) in (\"\")"=w245) -> ("States Out"=w244:string)  [unwired: 14 in]
      }
      frame "---------- Macro ----------" {
        # "Do not put any code in this frame.\n(It is a separator no-op. You can make a copy of this frame to create a new Macro frame)"
        n115 = call <vilib>:"Add State(s) to Queue__JKI_lib_State_Machine.vi"("State(s) in (\"\")"=w315) -> ("States Out"=w314:string)  [unwired: 14 in]
      }
      frame "Macro: Initialize" {
        w317 = "Data: Initialize\nInitialize Core Data\n\nMap: Create\n\nUI: Refresh Connection Status\nUI: Initialize\nUI: Front Panel State >> Open\nSim: Create Stop Event\nMacro: MQTTConnect"  # Data: Initialize Initialize Core Data  Map: Create  UI: Refresh Connection Status UI: Initialize UI: Front Panel State >> Open Sim: Create Stop Event Macro: MQTTConnect
        # "Initialization Macro\n(This is called once, when the VI starts)"
        n116 = call <vilib>:"Add State(s) to Queue__JKI_lib_State_Machine.vi"("State(s) in Front (\"\")"=w317, "State(s) in (\"\")"=w321) -> ("States Out"=w320:string)  [unwired: 13 in]
      }
      frame "Macro: MQTTConnect" {
        n117 = call <vilib>:"Add State(s) to Queue__JKI_lib_State_Machine.vi"("State(s) in Front (\"\")"="MQTT: Create Client\nMQTT: Register for Events\nMQTT: Connect", "State(s) in (\"\")"=w327) -> ("States Out"=w326:string)  [unwired: 13 in]
      }
      frame "Macro: onConnection" {
        n118 = call <vilib>:"Add State(s) to Queue__JKI_lib_State_Machine.vi"("State(s) in Front (\"\")"="MQTT: Subscribe\nMQTT: PublishConnectionMessage\nMQTT: PublishZoneList", "State(s) in (\"\")"=w333) -> ("States Out"=w332:string)  [unwired: 13 in]
      }
      frame "Macro: Handle Car State Msg" {
        n119 = call <vilib>:"Add State(s) to Queue__JKI_lib_State_Machine.vi"("State(s) in Front (\"\")"="MQTT: Handle Car State Msg\nMQTT: PublishZoneUpdates", "State(s) in (\"\")"=w339) -> ("States Out"=w338:string)  [unwired: 13 in]
      }
      frame "Macro: Handle Car Position Msg" {
        n120 = call <vilib>:"Add State(s) to Queue__JKI_lib_State_Machine.vi"("State(s) in Front (\"\")"="MQTT: Handle Car Position Msg\n//MQTT: PublishZoneUpdates", "State(s) in (\"\")"=w345) -> ("States Out"=w344:string)  [unwired: 13 in]
      }
      frame "Macro: Handle Car Disconnection Msg" {
        n121 = call <vilib>:"Add State(s) to Queue__JKI_lib_State_Machine.vi"("State(s) in Front (\"\")"="MQTT: Handle Car Disconnection Msg\nMQTT: PublishZoneUpdates", "State(s) in (\"\")"=w351) -> ("States Out"=w350:string)  [unwired: 13 in]
      }
      frame "Macro: Handle Will Msg" {
        n122 = call <vilib>:"Add State(s) to Queue__JKI_lib_State_Machine.vi"("State(s) in Front (\"\")"="MQTT: Handle Will Msg\nMQTT: PublishZoneUpdates", "State(s) in (\"\")"=w357) -> ("States Out"=w356:string)  [unwired: 13 in]
      }
      frame "Macro: Compute Now" {
        n123 = call <vilib>:"Add State(s) to Queue__JKI_lib_State_Machine.vi"("State(s) in Front (\"\")"="UI: Refresh Status Table\nMap: Compute Traffic\nMap: Display Traffic Update", "State(s) in (\"\")"=w363) -> ("States Out"=w362:string)  [unwired: 13 in]
      }
      frame "Macro: onDisconnection" {
        n124 = call <vilib>:"Add State(s) to Queue__JKI_lib_State_Machine.vi"("State(s) in (\"\")"=w368) -> ("States Out"=w367:string)  [unwired: 14 in]
      }
      frame "Macro: MQTTDisconnect" {
        n125 = call <vilib>:"Add State(s) to Queue__JKI_lib_State_Machine.vi"("State(s) in Front (\"\")"="MQTT: Unsubscribe\nMQTT: Unregister\nMQTT: PublishDisconnectionMessage\nMQTT: Disconnect\nMQTT: Destroy Client", "State(s) in (\"\")"=w374) -> ("States Out"=w373:string)  [unwired: 13 in]
      }
      frame "Macro: Exit" {
        # "Exit Macro\n(This is called once, when the VI exits)"
        n126 = Destroy User Event(user event=w375) -> (error out=w376:errorcluster)  [unwired: 1 in]
        n127 = Unbundle By Name(w385) -> ("Core.Close Panel on Exit?"=w384:bool)
        n128 = call <vilib>:"Clear Errors.vi"("error in (no error)"=w376) -> ()  [unwired: 5 in, 2 out]
        n129 = Select(t="UI: Front Panel State >> Close", s=w384, f="") -> (s? t:f=w381:string)
        n130 = call <vilib>:"Add State(s) to Queue__JKI_lib_State_Machine.vi"("State(s) in Front (\"\")"="Sim: Send Stop Signal\nMacro: MQTTDisconnect\nUI: Refresh Connection Status", "State(s) in (\"\")"=w381, "State(s) at Back (\"\")"="Data: Cleanup\nExit") -> ("States Out"=w379:string)  [unwired: 12 in]
        n131 = call <vilib>:"Add State(s) to Queue__JKI_lib_State_Machine.vi"("State(s) in Front (\"\")"=w379, "State(s) in (\"\")"=w388) -> ("States Out"=w387:string)  [unwired: 13 in]
      }
      frame "---------- Simulation ----------" {
        # "Simulation Separator\n(You can make a copy of, or modify, this frame)"
        n132 = call <vilib>:"Add State(s) to Queue__JKI_lib_State_Machine.vi"("State(s) in (\"\")"=w393) -> ("States Out"=w392:string)  [unwired: 14 in]
      }
      frame "Sim: Create Stop Event" {
        w397 = FALSE  # stop
        n133 = Create User Event(user event datatype=w397) -> (user event=w396:refnum<user-event>)  [unwired: 1 in, 1 out]
        n134 = Bundle By Name(cluster=w395, "stop signal"=w396) -> (w394:T12)
        n135 = call <vilib>:"Add State(s) to Queue__JKI_lib_State_Machine.vi"("State(s) in (\"\")"=w401) -> ("States Out"=w400:string)  [unwired: 14 in]
      }
      frame "Sim: Destroy Stop Event" {
        n136 = Unbundle By Name(w403) -> ("stop signal"=w402:refnum<user-event>)
        n137 = Destroy User Event(user event=w402) -> ()  [unwired: 1 in, 1 out]
        n138 = call <vilib>:"Add State(s) to Queue__JKI_lib_State_Machine.vi"("State(s) in (\"\")"=w407) -> ("States Out"=w406:string)  [unwired: 14 in]
      }
      frame "Sim: Send Stop Signal" {
        n139 = Unbundle By Name(w410) -> ("stop signal"=w412:refnum<user-event>)
        n140 = Unbundle By Name(w410) -> ()  [unwired: 1 out]
        n141 = Generate User Event(user event=w412, event data cluster=TRUE ("event data")) -> ()  [unwired: 2 in, 2 out]
        n142 = Bundle By Name(cluster=w410, "Clones"=string[] []) -> (w409:T12)
        n143 = call <vilib>:"Add State(s) to Queue__JKI_lib_State_Machine.vi"("State(s) in (\"\")"=w416) -> ("States Out"=w415:string)  [unwired: 14 in]
      }
      frame "Sim: Generate New Car" {
        n144 = Unbundle By Name(w421) -> ("stop signal"=w423:refnum<user-event>, "project namespace"=w422:string)
        n145 = vi-ref "Simulated Car Client.vi"() -> (w425:refnum<vi>)
        n146 = property class="VI Interface Type 0"(reference=w425) -> (reference out=w427:refnum<vi>, "Name"=w426:string)  [unwired: 1 in, 1 out]
        n147 = for {
          N: "# Cars" -> [_]
          tunnel: w426 -> [w443]
          tunnel: w427 -> [w442]
          tunnel: w423 -> [w441]
          shift-right: [w436] -> _
          shift-left: _ -> [w438]
          tunnel: w422 -> [w435]
          tunnel: [w432] -> w417 mode=indexing
          n148 = Open VI Reference(type specifier VI Refnum (for type only)=w442, vi path=w443, options=192) -> (vi reference=w434:refnum<vi>)  [unwired: 3 in, 1 out]
          n149 = Format Into String(format string="Client%06d", w438) -> (resulting string=w440:string)  [unwired: 2 in, 1 out]
          n150 = property class="VI Interface Type 0"(reference=w434) -> (reference out=w433:refnum<vi>, "Clone Name"=w432:string)  [unwired: 1 in, 1 out]
          n151 = Increment(x=w438) -> (x+1=w437:u32)
          n152 = To Unsigned Long Integer(number=w437) -> (unsigned 32bit integer=w436:u32)
          n153 = call-by-ref "Start Asynchronous Call"(reference=w433, "stop signal"=w441, "project namespace"=w435, "Client Name"=w440) -> ()  [unwired: 10 in, 2 out]
        }
        n154 = Unbundle By Name(w421) -> ("Clones"=w419:string[])
        n155 = Build Array (concatenate)(w419, w417) -> (w418:string[])
        n156 = Bundle By Name(cluster=w421, "Clones"=w418) -> (w420:T12)
        n157 = call <vilib>:"Add State(s) to Queue__JKI_lib_State_Machine.vi"("State(s) in (\"\")"=w431) -> ("States Out"=w430:string)  [unwired: 14 in]
      }
      frame "---------- Requests ----------" {
        # "Handling Requests\n(You can make a copy of, or modify, this frame)"
        n158 = call <vilib>:"Add State(s) to Queue__JKI_lib_State_Machine.vi"("State(s) in (\"\")"=w449) -> ("States Out"=w448:string)  [unwired: 14 in]
      }
      frame "Request: Handle Incoming" {
        n159 = Unbundle By Name(w451) -> ("Client"=w456:refnum<class "Client.lvclass">, "AppMessage"=w457:refnum<class "PUBLISH.lvclass">)
        n160 = Unbundle By Name(w451) -> ("TrafficMap"=w450:refnum<class "TrafficMap.lvclass">)
        n161 = call "Decode Publish Packet.vim"("Payload type"=T3 {"request"="", "reply-to"=""} ("Request Payload"), "PUBLISH"=w457, "Client in"=w456) -> ("Payload"=w454:T3, "Client out"=w455:refnum<class "Client.lvclass">)  [unwired: 5 in, 2 out]
        n162 = Unbundle By Name(w454) -> ("reply-to"=w452:string, "request"=w453:string)
        n163 = case shown="\"map\"" w453 {
          selector: w453 -> [w467 w473 w479]
          tunnel: [w468 w474 w480] -> w459
          tunnel: w450 -> [_ w471 w477]
          frame Default {
            w469 = "Unhandled Request"  # response
            n164 = Bundle(cluster=T4 {"request"="", "reply"=variant(string "")}, "request"=w467, "reply"=w469) -> (w468:T4)
          }
          frame "list-zones" {
            n165 = call "List Zones.vi"("TrafficMap in"=w471) -> ("Zones"=w475:string[])  [unwired: 7 in, 3 out]
            n166 = Bundle(cluster=T4 {"request"="", "reply"=variant(string "")}, "request"=w473, "reply"=w475) -> (w474:T4)
          }
          frame "map" {
            n167 = call "Read Map.vi"("TrafficMap in"=w477) -> ("Map"=w476:u16[][])  [unwired: 8 in, 2 out]
            n168 = Bundle(cluster=T4 {"request"="", "reply"=variant(string "")}, "request"=w479, "reply"=w476) -> (w480:T4)
          }
        }
        n169 = call <vilib>:"Publish.vi"("error in (no error)"=w461, "Payload"=w459, "Topic Name (empty: Payload name)"=w452, "Client in"=w455) -> ("error out"=w460:errorcluster, "Client out"=w462:refnum<class "Client.lvclass">)  [unwired: 5 in, 1 out]
        n170 = Bundle By Name(cluster=w451, "Client"=w462) -> (w464:T12)
        n171 = call <vilib>:"Add State(s) to Queue__JKI_lib_State_Machine.vi"("State(s) in (\"\")"=w466) -> ("States Out"=w465:string)  [unwired: 14 in]
      }
      frame "---------- Map ----------" {
        # "Map Separator\n(You can make a copy of, or modify, this frame)"
        n172 = call <vilib>:"Add State(s) to Queue__JKI_lib_State_Machine.vi"("State(s) in (\"\")"=w485) -> ("States Out"=w484:string)  [unwired: 14 in]
      }
      frame "Map: Create" {
        # "Map Separator\n(You can make a copy of, or modify, this frame)"
        n173 = call "Create TrafficMap.vi"("Zones"=string[] ["A", "B", "C", "D"]) -> ("TrafficMap"=w488:refnum<class "TrafficMap.lvclass">)  [unwired: 9 in, 1 out]
        n174 = Bundle By Name(cluster=w487, "TrafficMap"=w488) -> (w486:T12)
        n175 = call <vilib>:"Add State(s) to Queue__JKI_lib_State_Machine.vi"("State(s) in (\"\")"=w493) -> ("States Out"=w492:string)  [unwired: 14 in]
      }
      frame "Map: Compute Traffic" {
        # "Update Zones"
        n176 = Unbundle By Name(w511) -> ("TrafficMap"=w503:refnum<class "TrafficMap.lvclass">, "CarPool"=w504:refnum<class "CarPool.lvclass">)
        n177 = call "List Cars.vi"("CarPool in"=w504) -> ("Instances"=w512:refnum<class "Car.lvclass">[])  [unwired: 7 in, 3 out]
        n178 = call "Reset Counts.vi"("TrafficMap in"=w503) -> ("TrafficMap out"=w502:refnum<class "TrafficMap.lvclass">)  [unwired: 9 in, 1 out]
        n179 = call "List Zones.vi"("TrafficMap in"=w502) -> ("Instances"=w505:refnum<class "Zone.lvclass">[], "Zones"=w506:string[], "TrafficMap out"=w509:refnum<class "TrafficMap.lvclass">)  [unwired: 7 in, 1 out]
        n180 = for {
          tunnel: w512 -> [w525] mode=indexing
          shift-right: [w529] -> w507
          shift-left: w505 -> [w530]
          shift-right: [w521] -> w508
          shift-left: w506 -> [w521]
          tunnel: w500 -> [_]
          n181 = call "Read Position.vi"("Car in"=w525) -> ("Position"=w531:string)  [unwired: 8 in, 2 out]
          n182 = call "Read car state.vi"("Car in"=w525) -> ("car state"=w524:T5)  [unwired: 8 in, 2 out]
          n183 = Search 1D Array(1D array=w521, element=w531) -> (index of element=w528:i32)  [unwired: 1 in]
          n184 = Equal?(x=w524, y=Car_State_--_enum."driving") -> (x = y?=w523:bool)
          n185 = Index Array(array=w530, index=w528) -> (element=w527:refnum<class "Zone.lvclass">)
          n186 = call "Add One Car.vi"("Driving"=w523, "Zone in"=w527) -> ("Zone out"=w526:refnum<class "Zone.lvclass">)  [unwired: 8 in, 1 out]
          n187 = Replace Array Subset(array=w530, new element=w526, index=w528) -> (w529:refnum<class "Zone.lvclass">[])
        }
        n188 = for {
          tunnel: w508 -> [w519] mode=indexing
          tunnel: w507 -> [w518] mode=indexing
          shift-right: [w517] -> w501
          shift-left: w509 -> [w520]
          n189 = call "Update Zone.vi"("Zone Instance"=w518, "Zone Name"=w519, "TrafficMap in"=w520) -> ("TrafficMap out"=w517:refnum<class "TrafficMap.lvclass">)  [unwired: 7 in, 1 out]
        }
        n190 = feedback #2() -> (w499:refnum<class "TrafficMap.lvclass">)
        n191 = call "Compute Traffic Heat Map.vi"("TrafficMap in"=w501) -> ("TrafficMap out"=w498:refnum<class "TrafficMap.lvclass">)  [unwired: 8 in, 2 out]
        n192 = Not Equal?(x=w498, y=w499) -> (x != y?=w497:bool)
        n193 = feedback-in #2(w498) -> ()
        n194 = Bundle By Name(cluster=w511, "TrafficMap"=w498) -> (w510:T12)
        n195 = Select(t="MQTT: PublishZoneUpdates", s=w497, f="") -> (s? t:f=w494:string)
        n196 = call <vilib>:"Add State(s) to Queue__JKI_lib_State_Machine.vi"("State(s) in Front (\"\")"=w494, "State(s) in (\"\")"=w516) -> ("States Out"=w515:string)  [unwired: 13 in]
      }
      frame "Map: Display Traffic Update" {
        n197 = Unbundle By Name(w536) -> ("TrafficMap"=w535:refnum<class "TrafficMap.lvclass">)  [unwired: 1 out]
        n198 = call "Read Map.vi"("TrafficMap in"=w535) -> ("Map"=w534:u16[][])  [unwired: 8 in, 2 out]
        "Map" <- w534
        n199 = Array Size(array=w534) -> (size(s)=w533:i32[])
        n200 = Multiply Array Elements(1:w533) -> (0:w532:i32)
        n201 = Reshape Array(w534, w532) -> ()  [unwired: 1 out]
        n202 = call <vilib>:"Add State(s) to Queue__JKI_lib_State_Machine.vi"("State(s) in (\"\")"=w540) -> ("States Out"=w539:string)  [unwired: 14 in]
      }
      frame "---------- MQTT ----------" {
        # "MQTT Separator\n(You can make a copy of, or modify, this frame)"
        n203 = call <vilib>:"Add State(s) to Queue__JKI_lib_State_Machine.vi"("State(s) in (\"\")"=w545) -> ("States Out"=w544:string)  [unwired: 14 in]
      }
      frame "MQTT: Create Client" {
        # "Set JKI-JSON as the Serializer Class"
        n204 = call <vilib>:"Create MQTT Client.vi"("error in (no error)"=w553, "ID (empty:generate new)"="TrafficHub") -> ("error out"=w548:errorcluster, "Client out"=w551:refnum<class "Client.lvclass">)  [unwired: 8 in]
        n205 = call <vilib>:"Set Serializer.vi"("error in (no error)"=w548, "Serializer (default: Flattened String)"=refnum<class "Serializer.JKI-JSON.lvclass"> refnum ("Serializer.JKI-JSON.lvclass"), "MQTT_Base"=w551) -> ("error out"=w547:errorcluster, "MQTT_Base out"=w550:refnum<class "Client.lvclass">)  [unwired: 7 in]
        n206 = Bundle By Name(cluster=w555, "Client"=w550) -> (w554:T12)
        n207 = call <vilib>:"Add State(s) to Queue__JKI_lib_State_Machine.vi"("State(s) in (\"\")"=w557) -> ("States Out"=w556:string)  [unwired: 14 in]
      }
      frame "MQTT: Register for Events" {
        n208 = Unbundle By Name(w566) -> ("Client"=w564:refnum<class "Client.lvclass">)
        n209 = call <vilib>:"Read Public Events.vi"("error in (no error)"=w562, "Client in"=w564) -> ("error out"=w560:errorcluster, "Client Public Events"=w565:T16, "Client out"=w563:refnum<class "Client.lvclass">)  [unwired: 7 in]
        n210 = register-events(error in=w560, w565, w558) -> (reference out=w561:refnum<event-registration>, error out=w559:errorcluster)  [unwired: 1 in]
        n211 = Bundle By Name(cluster=w566, "Client"=w563) -> (w567:T12)
        n212 = call <vilib>:"Add State(s) to Queue__JKI_lib_State_Machine.vi"("State(s) in (\"\")"=w569) -> ("States Out"=w568:string)  [unwired: 14 in]
      }
      frame "MQTT: Connect" {
        n213 = Unbundle By Name(w590) -> ("server address"=w583:string, "Client"=w586:refnum<class "Client.lvclass">, "project namespace"=w575:string, "Client Name"=w574:string)
        n214 = call <vilib>:"Start.vi"("error in (no error)"=w585, "MQTT_Base in"=w586) -> ("error out"=w588:errorcluster, "MQTT_Base out"=w587:refnum<class "Client.lvclass">)  [unwired: 7 in, 1 out]
        n215 = call <vilib>:"Flatten To JSON String.vi"("Variant"=cluster{"message":string} {"message"="unexpected disconnection"}) -> ("JSON String"=w570:string)  [unwired: 9 in, 1 out]
        n216 = Format Into String(format string="%s/%s/will", w575, w574) -> (resulting string=w576:string)  [unwired: 2 in, 1 out]
        n217 = Bundle By Name(cluster=T6 {"Reserved"=FALSE, "Clean Session"=FALSE, "Will Flag"=FALSE, "Will QoS 1"=FALSE, "Will QoS 2"=FALSE, "Will Retain"=FALSE, "Password Flag"=FALSE, "User Name Flag"=FALSE} ("Connect Flags"), "Will Flag"=TRUE) -> (w578:T6)
        n218 = Bundle By Name(cluster=T7 {"Will Topic"="", "Will Message"="", "Username"="", "Password"=""} ("Payload"), "Will Topic"=w576, "Will Message"=w570) -> (w572:T7)
        n219 = call <vilib>:"Connect to Server.vi"("Connect Flags"=w578, "Keep Alive (s)"=u16 3600, "Payload"=w572, "error in (no error)"=w588, "address (localhost)"=w583, "Client in"=w587) -> ("error out"=w584:errorcluster, "Client out"=w582:refnum<class "Client.lvclass">)  [unwired: 2 in, 2 out]
        n220 = Bundle By Name(cluster=w590, "Client"=w582) -> (w591:T12)
        n221 = call <vilib>:"Add State(s) to Queue__JKI_lib_State_Machine.vi"("State(s) in (\"\")"=w593) -> ("States Out"=w592:string)  [unwired: 14 in]
      }
      frame "MQTT: Check Connection" {
        n222 = Unbundle By Name(w597) -> ("Client"=w598:refnum<class "Client.lvclass">)
        n223 = call <vilib>:"isConnected.vi"("error in (no error)"=w595, "Client in"=w598) -> ("error out"=w594:errorcluster, "connected"=w601:bool)  [unwired: 7 in, 1 out]
        n224 = Select(t="", s=w601, f="UI: Refresh Connection Status") -> (s? t:f=w596:string)
        n225 = call <vilib>:"Add State(s) to Queue__JKI_lib_State_Machine.vi"("State(s) in Front (\"\")"=w596, "State(s) in (\"\")"=w604) -> ("States Out"=w603:string)  [unwired: 13 in]
      }
      frame "MQTT: Subscribe" {
        n226 = Unbundle By Name(w614) -> ("project namespace"=w611:string, "Subscription"=w610:string, "Client"=w609:refnum<class "Client.lvclass">)
        n227 = Format Into String(format string="%s/%s", w611, w610) -> (resulting string=w605:string)  [unwired: 2 in, 1 out]
        n228 = call <vilib>:"Subscribe (SingleTopic).vi"("error in (no error)"=w607, "Topic Filter"=w605, "MQTT_Base in"=w609) -> ("error out"=w606:errorcluster, "MQTT_Base out"=w608:refnum<class "Client.lvclass">)  [unwired: 7 in]
        n229 = Bundle By Name(cluster=w614, "Client"=w608) -> (w615:T12)
        n230 = call <vilib>:"Add State(s) to Queue__JKI_lib_State_Machine.vi"("State(s) in (\"\")"=w617) -> ("States Out"=w616:string)  [unwired: 14 in]
      }
      frame "MQTT: Unsubscribe" {
        n231 = Unbundle By Name(w627) -> ("project namespace"=w620:string, "Subscription"=w618:string, "Client"=w625:refnum<class "Client.lvclass">)
        n232 = Format Into String(format string="%s/%s", w620, w618) -> (resulting string=w619:string)  [unwired: 2 in, 1 out]
        n233 = call <vilib>:"Unsubscribe (SingleTopic).vi"("error in (no error)"=w623, "Topic Filter"=w619, "MQTT_Base in"=w625) -> ("error out"=w622:errorcluster, "MQTT_Base out"=w624:refnum<class "Client.lvclass">)  [unwired: 7 in]
        n234 = Bundle By Name(cluster=w627, "Client"=w624) -> (w628:T12)
        n235 = call <vilib>:"Add State(s) to Queue__JKI_lib_State_Machine.vi"("State(s) in (\"\")"=w630) -> ("States Out"=w629:string)  [unwired: 14 in]
      }
      frame "MQTT: PublishOwnState" {
        n236 = Unbundle By Name(w641) -> ("project namespace"=w636:string, "Client Name"=w635:string, "Client"=w638:refnum<class "Client.lvclass">)
        n237 = Format Into String(format string="%s/users/%s/last-update", w636, w635) -> (resulting string=w634:string)  [unwired: 2 in, 1 out]
        n238 = call "Formatted Timestamp.vi"() -> ("String Formatted timestamp"=w631:string)  [unwired: 11 in]
        n239 = call <vilib>:"Publish.vi"("error in (no error)"=w633, "Payload"=w631, "Topic Name (empty: Payload name)"=w634, "Client in"=w638) -> ("error out"=w632:errorcluster, "Client out"=w639:refnum<class "Client.lvclass">)  [unwired: 5 in, 1 out]
        n240 = Bundle By Name(cluster=w641, "Client"=w639) -> (w642:T12)
        n241 = call <vilib>:"Add State(s) to Queue__JKI_lib_State_Machine.vi"("State(s) in (\"\")"=w644) -> ("States Out"=w643:string)  [unwired: 14 in]
      }
      frame "MQTT: Handle App Message" {
        n242 = Unbundle By Name(w645) -> ("Client Name"=w646:string, "Client"=w653:refnum<class "Client.lvclass">, "AppMessage"=w649:refnum<class "PUBLISH.lvclass">)
        n243 = call <vilib>:"getTopicName.vi"("PUBLISH in"=w649) -> ("Topic"=w652:string, "PUBLISH out"=w654:refnum<class "PUBLISH.lvclass">)  [unwired: 8 in, 1 out]
        "Topic" <- w652
        n244 = call <vilib>:"Read Payload.vi"("ControlPacket in"=w649) -> ("Payload"=w648:u8[])  [unwired: 9 in, 1 out]
        n245 = call "topic_to_Array.vi"("Topic"=w652) -> ("Topic (Array)"=w656:string[])  [unwired: 10 in]
        n246 = Byte Array To String(unsigned byte array=w648) -> (string=→"Raw Packet String":string)
        n247 = Delete From Array(array=w656) -> (deleted portion=w655:string, array with subset deleted=w651:string[])  [unwired: 2 in]
        n248 = case shown="\"state\"" w655 {
          tunnel: w654 -> [w662 w674 w679 _ _ _ _]
          tunnel: w653 -> [w663 w675 w680 _ _ _ _]
          tunnel: w651 -> [_ w670 w684 _ _ _ _]
          tunnel: [_ w676 _ "Macro: Handle Car State Msg" "Macro: Handle Car Position Msg" "Macro: Handle Car Disconnection Msg" "Macro: Handle Will Msg"] -> w650
          tunnel: w646 -> [_ w671 w681 _ _ _ _]
          frame Default {
            n249 = call "Decode Publish Packet.vim"("PUBLISH"=w662, "Client in"=w663) -> ("Payload"=→"Payload":variant)  [unwired: 6 in, 3 out]
          }
          frame "request" {
            n250 = Index Array(array=w670, index #1=1 ("index"), index #2=2 ("index")) -> (element #1=w668:string, element #2=w672:string)
            n251 = Equal?(x="traffic-data", y=w668) -> (x = y?=w666:bool)
            n252 = Equal?(x=w671, y=w672) -> (x = y?=w665:bool)
            n253 = Compound Arithmetic op=OR(w666, w665) -> (w664:bool)
            n254 = case shown="True" w664 {
              tunnel: [_ "Request: Handle Incoming"] -> w676
              tunnel: w675 -> [_ _]
              tunnel: w674 -> [_ _]
              frame False {
              }
              frame True {
              }
            }
          }
          frame "inbox" {
            n255 = Index Array(array=w684, index=2) -> (element=w682:string)
            n256 = Equal?(x=w681, y=w682) -> (x = y?=w678:bool)
            n257 = case shown="True" w678 {
              tunnel: w680 -> [_ w689]
              tunnel: w679 -> [_ w688]
              frame False {
              }
              frame True {
                n258 = call "Decode Publish Packet.vim"("Payload type"=T4 {"request"="", "reply"=variant} ("Response Payload"), "PUBLISH"=w688, "Client in"=w689) -> ("Payload"=w687:T4)  [unwired: 5 in, 3 out]
                n259 = Unbundle(w687) -> ("request"=w686:string, "reply"=w685:variant)
                n260 = case shown="\"list-zones\"" w686 {
                  tunnel: w685 -> [_ w695]
                  frame "False", Default {
                  }
                  frame "list-zones" {
                    w692 = string[] []
                    n261 = call <vilib>:"Adapt To Type.vi"("Type and Defaults"=w692, "Variant in"=w695) -> ("error out"=w694:errorcluster, "Variant out"=w693:variant)  [unwired: 8 in]
                    n262 = Variant To Data(error in=w694, type=w692, Variant=w693) -> (data=→"Zones":string[])  [unwired: 1 out]
                  }
                }
              }
            }
          }
          frame "state" {
          }
          frame "position" {
          }
          frame "disconnect" {
          }
          frame "will" {
          }
        }
        n263 = call <vilib>:"Add State(s) to Queue__JKI_lib_State_Machine.vi"("State(s) in Front (\"\")"=w650, "State(s) in (\"\")"=w660) -> ("States Out"=w659:string)  [unwired: 13 in]
      }
      frame "MQTT: Handle Car State Msg" {
        n264 = Unbundle By Name(w721) -> ("Client"=w715:refnum<class "Client.lvclass">, "AppMessage"=w714:refnum<class "PUBLISH.lvclass">, "CarPool"=w704:refnum<class "CarPool.lvclass">)
        n265 = call "Decode Publish Packet.vim"("Payload type"="", "PUBLISH"=w714, "Client in"=w715) -> ("Payload"=w711:string, "Topic"=w718:string, "Client out"=w713:refnum<class "Client.lvclass">)  [unwired: 5 in, 1 out]
        n266 = call "topic_to_Array.vi"("Topic"=w718) -> ("Topic (Array)"=w712:string[])  [unwired: 10 in]
        n267 = Delete From Array(array=w712, index=2) -> (deleted portion=w701:string)  [unwired: 1 in, 1 out]
        n268 = call "Get Car Instance.vi"("Car Name"=w701, "CarPool in"=w704) -> ("Car"=w702:refnum<class "Car.lvclass">, "CarPool out"=w705:refnum<class "CarPool.lvclass">)  [unwired: 6 in, 2 out]
        n269 = call "Read car state.vi"("Car in"=w702) -> ("car state"=w710:T5, "Car out"=w707:refnum<class "Car.lvclass">)  [unwired: 8 in, 1 out]
        n270 = Scan From String(input string=w711, default 1=w710) -> (output 1=w709:T5)  [unwired: 3 in, 3 out]
        n271 = call "Write disconnected.vi"("disconnected"=FALSE, "Car in"=w707) -> ("Car out"=w706:refnum<class "Car.lvclass">)  [unwired: 8 in, 1 out]
        n272 = call "Write car state.vi"("car state"=w709, "Car in"=w706) -> ("Car out"=w700:refnum<class "Car.lvclass">)  [unwired: 8 in, 1 out]
        n273 = call "Update Car Instance.vi"("Car Name"=w701, "Car"=w700, "CarPool in"=w705) -> ("CarPool out"=w703:refnum<class "CarPool.lvclass">)  [unwired: 7 in, 1 out]
        n274 = Bundle By Name(cluster=w721, "Client"=w713, "CarPool"=w703) -> (w722:T12)
        n275 = call <vilib>:"Add State(s) to Queue__JKI_lib_State_Machine.vi"("State(s) in (\"\")"=w724) -> ("States Out"=w723:string)  [unwired: 14 in]
      }
      frame "MQTT: Handle Car Position Msg" {
        n276 = Unbundle By Name(w750) -> ("Client"=w744:refnum<class "Client.lvclass">, "AppMessage"=w743:refnum<class "PUBLISH.lvclass">, "TrafficMap"=w739:refnum<class "TrafficMap.lvclass">, "CarPool"=w730:refnum<class "CarPool.lvclass">)
        n277 = call "Decode Publish Packet.vim"("Payload type"="", "PUBLISH"=w743, "Client in"=w744) -> ("Payload"=w735:string, "Topic"=w747:string, "Client out"=w742:refnum<class "Client.lvclass">)  [unwired: 5 in, 1 out]
        n278 = call "List Zones.vi"("TrafficMap in"=w739) -> ("Zones"=w738:string[])  [unwired: 7 in, 3 out]
        n279 = call "topic_to_Array.vi"("Topic"=w747) -> ("Topic (Array)"=w741:string[])  [unwired: 10 in]
        n280 = Delete From Array(array=w741, index=2) -> (deleted portion=w729:string)  [unwired: 1 in, 1 out]
        n281 = call "Get Car Instance.vi"("Car Name"=w729, "CarPool in"=w730) -> ("Car"=w726:refnum<class "Car.lvclass">, "CarPool out"=w728:refnum<class "CarPool.lvclass">)  [unwired: 6 in, 2 out]
        n282 = Search 1D Array(1D array=w738, element=w735) -> (index of element=w737:i32)  [unwired: 1 in]
        n283 = Greater Or Equal To 0?(x=w737) -> (x >= 0?=w736:bool)
        n284 = call "Write disconnected.vi"("disconnected"=FALSE, "Car in"=w726) -> ("Car out"=w731:refnum<class "Car.lvclass">)  [unwired: 8 in, 1 out]
        n285 = call "Read Position.vi"("Car in"=w731) -> ("Position"=w734:string, "Car out"=w740:refnum<class "Car.lvclass">)  [unwired: 8 in, 1 out]
        n286 = Select(t=w735, s=w736, f=w734) -> (s? t:f=w733:string)
        n287 = call "Write Position.vi"("Position"=w733, "Car in"=w740) -> ("Car out"=w725:refnum<class "Car.lvclass">)  [unwired: 8 in, 1 out]
        n288 = call "Update Car Instance.vi"("Car Name"=w729, "Car"=w725, "CarPool in"=w728) -> ("CarPool out"=w727:refnum<class "CarPool.lvclass">)  [unwired: 7 in, 1 out]
        n289 = Bundle By Name(cluster=w750, "Client"=w742, "CarPool"=w727) -> (w751:T12)
        n290 = call <vilib>:"Add State(s) to Queue__JKI_lib_State_Machine.vi"("State(s) in (\"\")"=w753) -> ("States Out"=w752:string)  [unwired: 14 in]
      }
      frame "MQTT: Handle Car Disconnection Msg" {
        n291 = Unbundle By Name(w776) -> ("Client"=w771:refnum<class "Client.lvclass">, "AppMessage"=w770:refnum<class "PUBLISH.lvclass">, "CarPool"=w756:refnum<class "CarPool.lvclass">)  [unwired: 1 out]
        n292 = call "Decode Publish Packet.vim"("Payload type"=T8 {"timestamp"=""} ("Disconnect payload"), "PUBLISH"=w770, "Client in"=w771) -> ("Payload"=w767:T8, "Topic"=w773:string, "Client out"=w769:refnum<class "Client.lvclass">)  [unwired: 5 in, 1 out]
        n293 = call "topic_to_Array.vi"("Topic"=w773) -> ("Topic (Array)"=w768:string[])  [unwired: 10 in]
        n294 = Unbundle(w767) -> ("timestamp"=w764:string)
        n295 = Delete From Array(array=w768, index=2) -> (deleted portion=w757:string)  [unwired: 1 in, 1 out]
        n296 = call "Get Car Instance.vi"("Car Name"=w757, "CarPool in"=w756) -> ("Car"=w755:refnum<class "Car.lvclass">, "CarPool out"=w759:refnum<class "CarPool.lvclass">)  [unwired: 6 in, 2 out]
        n297 = call "Write disconnected.vi"("disconnected"=TRUE, "Car in"=w755) -> ("Car out"=w765:refnum<class "Car.lvclass">)  [unwired: 8 in, 1 out]
        n298 = Scan From String(format string="%<%Y%m%d-%H:%M:%S>T", input string=w764, default 1=timestamp(0 s since 1904-01-01)) -> (output 1=w762:timestamp)  [unwired: 2 in, 3 out]
        n299 = call "Write disconnection time.vi"("disconnection time"=w762, "Car in"=w765) -> ("Car out"=w754:refnum<class "Car.lvclass">)  [unwired: 8 in, 1 out]
        n300 = call "Update Car Instance.vi"("Car Name"=w757, "Car"=w754, "CarPool in"=w759) -> ("CarPool out"=w758:refnum<class "CarPool.lvclass">)  [unwired: 7 in, 1 out]
        n301 = Bundle By Name(cluster=w776, "Client"=w769, "CarPool"=w758) -> (w777:T12)
        n302 = call <vilib>:"Add State(s) to Queue__JKI_lib_State_Machine.vi"("State(s) in (\"\")"=w779) -> ("States Out"=w778:string)  [unwired: 14 in]
      }
      frame "MQTT: Handle Will Msg" {
        n303 = Unbundle By Name(w799) -> ("Client"=w794:refnum<class "Client.lvclass">, "AppMessage"=w793:refnum<class "PUBLISH.lvclass">, "CarPool"=w782:refnum<class "CarPool.lvclass">)  [unwired: 1 out]
        n304 = call "Decode Publish Packet.vim"("Payload type"=T9 {"message"="unexpected disconnection"} ("Will Payload"), "PUBLISH"=w793, "Client in"=w794) -> ("Payload"=w790:T9, "Topic"=w796:string, "Client out"=w792:refnum<class "Client.lvclass">)  [unwired: 5 in, 1 out]
        n305 = call "topic_to_Array.vi"("Topic"=w796) -> ("Topic (Array)"=w791:string[])  [unwired: 10 in]
        n306 = Unbundle(w790) -> ()  [unwired: 1 out]
        n307 = Delete From Array(array=w791, index=2) -> (deleted portion=w781:string)  [unwired: 1 in, 1 out]
        n308 = call "Get Car Instance.vi"("Car Name"=w781, "CarPool in"=w782) -> ("Car"=w783:refnum<class "Car.lvclass">, "CarPool out"=w785:refnum<class "CarPool.lvclass">)  [unwired: 6 in, 2 out]
        n309 = call "Write disconnected.vi"("disconnected"=TRUE, "Car in"=w783) -> ("Car out"=w788:refnum<class "Car.lvclass">)  [unwired: 8 in, 1 out]
        n310 = Get Date/Time In Seconds() -> (seconds since 1Jan1904=w786:timestamp)
        n311 = call "Write disconnection time.vi"("disconnection time"=w786, "Car in"=w788) -> ("Car out"=w784:refnum<class "Car.lvclass">)  [unwired: 8 in, 1 out]
        n312 = call "Update Car Instance.vi"("Car Name"=w781, "Car"=w784, "CarPool in"=w785) -> ("CarPool out"=w780:refnum<class "CarPool.lvclass">)  [unwired: 7 in, 1 out]
        n313 = Bundle By Name(cluster=w799, "Client"=w792, "CarPool"=w780) -> (w800:T12)
        n314 = call <vilib>:"Add State(s) to Queue__JKI_lib_State_Machine.vi"("State(s) in (\"\")"=w802) -> ("States Out"=w801:string)  [unwired: 14 in]
      }
      frame "MQTT: Log Incoming Message" {
        n315 = Unbundle By Name(w807) -> ("Client"=w812:refnum<class "Client.lvclass">, "AppMessage"=w813:refnum<class "PUBLISH.lvclass">)
        n316 = call <vilib>:"getTopicName.vi"("PUBLISH in"=w813) -> ("Topic"=w809:string, "PUBLISH out"=w811:refnum<class "PUBLISH.lvclass">)  [unwired: 8 in, 1 out]
        n317 = call "topic_to_Array.vi"("Topic"=w809) -> ("Topic (Array)"=w810:string[])  [unwired: 10 in]
        n318 = Delete From Array(array=w810) -> (deleted portion=w808:string)  [unwired: 2 in, 1 out]
        n319 = case shown="Default" w808 {
          tunnel: w812 -> [w827 w833]
          tunnel: w811 -> [w826 w832]
          tunnel: w809 -> [w821 w835]
          tunnel: [w818 w834] -> w806
          frame "nb-cars" {
            n320 = call "Decode Publish Packet.vim"("Payload type"=u32 0 ("index (col)"), "PUBLISH"=w826, "Client in"=w827) -> ("Payload"=w819:u32)  [unwired: 5 in, 3 out]
            n321 = call <vilib>:"Read Fixed Header.vi"("ControlPacket in"=w826) -> ("Fixed Header"=w825:u8)  [unwired: 9 in, 1 out]
            n322 = call <vilib>:"ExtractFlagBits.vi"("Fixed Header"=w825) -> ("RETAIN"=w823:bool, "QoS"=w824:T17, "DUP"=w822:bool)  [unwired: 7 in, 1 out]
            n323 = Format Into String(format string="Message [Topic: %s, Payload: %d, QoS: %d, Retained: %s, Duplicate: %s]", w821, w819, w824, w823, w822) -> (resulting string=w818:string)  [unwired: 2 in, 1 out]
          }
          frame Default {
            n324 = call "Decode Publish Packet.vim"("PUBLISH"=w832, "Client in"=w833) -> ("Payload"=w831:variant)  [unwired: 6 in, 3 out]
            n325 = call <vilib>:"Read Fixed Header.vi"("ControlPacket in"=w832) -> ("Fixed Header"=w836:u8)  [unwired: 9 in, 1 out]
            n326 = call <userlib>:"Format Variant Into String__ogtk.vi"("Variant"=w831) -> ("Output String"=w830:string, "error out"=w829:errorcluster)  [unwired: 13 in]
            n327 = case shown="No Error" w829 {
              tunnel: w836 -> [w843 w851]
              tunnel: w835 -> [w839 w847]
              tunnel: [w837 w845] -> w834
              tunnel: w830 -> [w838 _]
              frame No Error {
                n328 = call <vilib>:"ExtractFlagBits.vi"("Fixed Header"=w843) -> ("RETAIN"=w841:bool, "QoS"=w842:T17, "DUP"=w840:bool)  [unwired: 7 in, 1 out]
                n329 = Format Into String(format string="Message [Topic: %s, Payload: %s, QoS: %d, Retained: %s, Duplicate: %s]", w839, w838, w842, w841, w840) -> (resulting string=w837:string)  [unwired: 2 in, 1 out]
              }
              frame Error {
                n330 = call <vilib>:"ExtractFlagBits.vi"("Fixed Header"=w851) -> ("RETAIN"=w849:bool, "QoS"=w850:T17, "DUP"=w848:bool)  [unwired: 7 in, 1 out]
                n331 = Format Into String(format string="Message [Topic: %s, Payload: %s, QoS: %d, Retained: %s, Duplicate: %s]", w847, "" ("format string"), w850, w849, w848) -> (resulting string=w845:string)  [unwired: 2 in, 1 out]
              }
            }
          }
        }
        "Last Incoming Message" <- w806
        n332 = feedback #3(u32 0 ("Messages Processed")) -> (w803:u32)
        "Messages Processed" <- w803
        n333 = Increment(x=w803) -> (x+1=w805:u32)
        n334 = feedback-in #3(w805) -> ()
        n335 = call <vilib>:"Add State(s) to Queue__JKI_lib_State_Machine.vi"("State(s) in (\"\")"=w817) -> ("States Out"=w816:string)  [unwired: 14 in]
      }
      frame "MQTT: RequestZoneList" {
        n336 = Unbundle By Name(w867) -> ("project namespace"=w855:string, "Client Name"=w854:string, "Client"=w864:refnum<class "Client.lvclass">)
        n337 = Format Into String(format string="%s/users/%s/inbox", w855, w854) -> (resulting string=w857:string)  [unwired: 2 in, 1 out]
        n338 = Format Into String(format string="%s/users/%s/request", w855, w854) -> (resulting string=w862:string)  [unwired: 2 in, 1 out]
        n339 = Bundle By Name(cluster=T3 {"request"="", "reply-to"=""} ("Request Payload"), "request"="list-zones" ("Request"), "reply-to"=w857) -> (w859:T3)
        n340 = call <vilib>:"Publish.vi"("error in (no error)"=w861, "Payload"=w859, "Topic Name (empty: Payload name)"=w862, "Client in"=w864) -> ("error out"=w860:errorcluster, "Client out"=w865:refnum<class "Client.lvclass">)  [unwired: 5 in, 1 out]
        n341 = Bundle By Name(cluster=w867, "Client"=w865) -> (w868:T12)
        n342 = call <vilib>:"Add State(s) to Queue__JKI_lib_State_Machine.vi"("State(s) in (\"\")"=w870) -> ("States Out"=w869:string)  [unwired: 14 in]
      }
      frame "MQTT: PublishZoneList" {
        # "LabVIEWDemo/traffic-data/zones"
        n343 = Unbundle By Name(w881) -> ("project namespace"=w873:string, "Client"=w878:refnum<class "Client.lvclass">, "TrafficMap"=w872:refnum<class "TrafficMap.lvclass">)  [unwired: 1 out]
        n344 = call "List Zones.vi"("TrafficMap in"=w872) -> ("Zones"=w871:string[])  [unwired: 7 in, 3 out]
        n345 = Format Into String(format string="%s/traffic-data/zones", w873) -> (resulting string=w876:string)  [unwired: 2 in, 1 out]
        n346 = call <vilib>:"Publish.vi"("error in (no error)"=w875, "Payload"=w871, "Topic Name (empty: Payload name)"=w876, "Client in"=w878) -> ("error out"=w874:errorcluster, "Client out"=w879:refnum<class "Client.lvclass">)  [unwired: 5 in, 1 out]
        n347 = Bundle By Name(cluster=w881, "Client"=w879) -> (w882:T12)
        n348 = call <vilib>:"Add State(s) to Queue__JKI_lib_State_Machine.vi"("State(s) in (\"\")"=w884) -> ("States Out"=w883:string)  [unwired: 14 in]
      }
      frame "MQTT: PublishZoneUpdates" {
        # "LabVIEWDemo/traffic-data/zones (list of traffic zones)\nLabVIEWDemo/traffic-data/zone/A/nb-cars (zone A cars in any states)\nLabVIEWDemo/traffic-data/zone/A/nb-drivers (zone A cars in Driving state)\nLabVIEWDemo/traffic-data/zone/B/nb-cars (zone B cars in any states)\nLabVIEWDemo/traffic-data/zone/B/nb-drivers (zone B cars in Driving state)"
        n349 = Unbundle By Name(w888) -> ("project namespace"=w891:string, "Client"=w892:refnum<class "Client.lvclass">, "TrafficMap"=w890:refnum<class "TrafficMap.lvclass">)  [unwired: 1 out]
        n350 = call "List Zones.vi"("error in (no error)"=w886, "TrafficMap in"=w890) -> ("error out"=w885:errorcluster, "Instances"=w887:refnum<class "Zone.lvclass">[], "Zones"=w889:string[])  [unwired: 6 in, 1 out]
        n351 = for {
          tunnel: w892 -> [w909]
          tunnel: w891 -> [w904]
          tunnel: w889 -> [w903] mode=indexing
          tunnel: w887 -> [w901] mode=indexing
          tunnel: [w897] -> _ mode=indexing
          n352 = call "Read Nb Cars.vi"("Zone in"=w901) -> ("Nb Cars"=w900:u32, "Zone out"=w899:refnum<class "Zone.lvclass">)  [unwired: 8 in, 1 out]
          n353 = call "Read Nb Cars Driving.vi"("Zone in"=w899) -> ("Nb Cars Driving"=w898:u32)  [unwired: 8 in, 2 out]
          n354 = Format Into String(format string="%s/traffic-data/zone/%s/nb-cars", w904, w903) -> (resulting string=w908:string)  [unwired: 2 in, 1 out]
          n355 = call <vilib>:"Publish.vi"("Payload"=w900, "Topic Name (empty: Payload name)"=w908, "Client in"=w909) -> ("error out"=w896:errorcluster, "Client out"=w907:refnum<class "Client.lvclass">)  [unwired: 6 in, 1 out]
          n356 = Format Into String(format string="%s/traffic-data/zone/%s/nb-drivers", w904, w903) -> (resulting string=w902:string)  [unwired: 2 in, 1 out]
          n357 = call <vilib>:"Publish.vi"("error in (no error)"=w896, "Payload"=w898, "Topic Name (empty: Payload name)"=w902, "Client in"=w907) -> ("error out"=w897:errorcluster)  [unwired: 5 in, 2 out]
        }
        n358 = call <vilib>:"Add State(s) to Queue__JKI_lib_State_Machine.vi"("State(s) in (\"\")"=w895) -> ("States Out"=w894:string)  [unwired: 14 in]
      }
      frame "MQTT: PublishConnectionMessage" {
        n359 = Unbundle By Name(w923) -> ("project namespace"=w918:string, "Client Name"=w917:string, "Client"=w920:refnum<class "Client.lvclass">, "Node type"=w913:T11)
        n360 = Format Into String(w913) -> (resulting string=w912:string)  [unwired: 3 in, 1 out]
        n361 = Format Into String(format string="%s/users/%s/connect", w918, w917) -> (resulting string=w916:string)  [unwired: 2 in, 1 out]
        n362 = Bundle(cluster=T10 {"Node type"=""} ("Connect payload"), "Node type"=w912) -> (w911:T10)
        n363 = call <vilib>:"Publish.vi"("error in (no error)"=w915, "Payload"=w911, "Topic Name (empty: Payload name)"=w916, "Client in"=w920) -> ("error out"=w914:errorcluster, "Client out"=w921:refnum<class "Client.lvclass">)  [unwired: 5 in, 1 out]
        n364 = Bundle By Name(cluster=w923, "Client"=w921) -> (w924:T12)
        n365 = call <vilib>:"Add State(s) to Queue__JKI_lib_State_Machine.vi"("State(s) in (\"\")"=w926) -> ("States Out"=w925:string)  [unwired: 14 in]
      }
      frame "MQTT: PublishDisconnectionMessage" {
        n366 = Unbundle By Name(w939) -> ("project namespace"=w934:string, "Client Name"=w933:string, "Client"=w936:refnum<class "Client.lvclass">)
        n367 = Format Into String(format string="%s/users/%s/disconnect", w934, w933) -> (resulting string=w932:string)  [unwired: 2 in, 1 out]
        n368 = call "Formatted Timestamp.vi"() -> ("String Formatted timestamp"=w928:string)  [unwired: 11 in]
        n369 = Bundle(cluster=T8 {"timestamp"=""} ("Disconnect payload"), "timestamp"=w928) -> (w927:T8)
        n370 = call <vilib>:"Publish.vi"("error in (no error)"=w931, "Payload"=w927, "Topic Name (empty: Payload name)"=w932, "Client in"=w936) -> ("error out"=w930:errorcluster, "Client out"=w937:refnum<class "Client.lvclass">)  [unwired: 5 in, 1 out]
        n371 = Bundle By Name(cluster=w939, "Client"=w937) -> (w940:T12)
        n372 = call <vilib>:"Add State(s) to Queue__JKI_lib_State_Machine.vi"("State(s) in (\"\")"=w942) -> ("States Out"=w941:string)  [unwired: 14 in]
      }
      frame "MQTT: Disconnect" {
        n373 = Unbundle By Name(w950) -> ("Client"=w948:refnum<class "Client.lvclass">)
        n374 = call <vilib>:"Disconnect from Server.vi"("error in (no error)"=w943, "Client in"=w948) -> ("error out"=w944:errorcluster, "Client out"=w947:refnum<class "Client.lvclass">)  [unwired: 7 in, 1 out]
        n375 = call <vilib>:"Stop.vi"("error in (no error)"=w944, "MQTT_Base in"=w947) -> ("error out"=w945:errorcluster, "MQTT_Base out"=w946:refnum<class "Client.lvclass">)  [unwired: 7 in, 1 out]
        n376 = Bundle By Name(cluster=w950, "Client"=w946) -> (w951:T12)
        n377 = call <vilib>:"Add State(s) to Queue__JKI_lib_State_Machine.vi"("State(s) in (\"\")"=w953) -> ("States Out"=w952:string)  [unwired: 14 in]
      }
      frame "MQTT: Unregister" {
        n378 = Unregister For Events(event registration refnum=w957, error in=w956) -> (error out=w955:errorcluster)
        n379 = call <vilib>:"Add State(s) to Queue__JKI_lib_State_Machine.vi"("State(s) in (\"\")"=w959) -> ("States Out"=w958:string)  [unwired: 14 in]
      }
      frame "MQTT: Destroy Client" {
        n380 = Unbundle By Name(w964) -> ("Client"=w963:refnum<class "Client.lvclass">)
        n381 = call-dynamic "Destroy.vi"("error in (no error)"=w962, "MQTT_Base in"=w963) -> ("error out"=w961:errorcluster)  [unwired: 8 in, 1 out]
        n382 = call <vilib>:"Add State(s) to Queue__JKI_lib_State_Machine.vi"("State(s) in (\"\")"=w966) -> ("States Out"=w965:string)  [unwired: 14 in]
      }
    }
  }
  n383 = while {
    tunnel: w2 -> [w969]
    stop <- w968 stop-if-true
    # "Recurrent Compute Message"
    n384 = event shown="[0] Timeout" {
      selector: _ -> [_]
      dyn-events: _ -> [_]
      timeout: 500 -> [_]
      tunnel: w969 -> [w972]
      tunnel: [w970] -> w968
      event Timeout {
        n385 = event-data() -> ()  [unwired: 1 in, 1 out]
        n386 = Generate User Event(user event=w972, event data cluster=TRUE ("event data")) -> (error out=w970:errorcluster)  [unwired: 2 in, 1 out]
      }
    }
  }
